vi "Process0.vi"(9 "process sync":refnum<notifier>, 11 "Main in":refnum<class "Main.lvclass">) -> ()   [LabVIEW 2019, in "Main.lvclass"]
doc: "Developed by Kevin Thompson\nkevin@thompsonengineering.net\n\nCopyright 2018\nThompson Engineering, LLC"
uses:
  Main.lvclass
  <vilib>/TELLC/SMQ/Add States to Queue using MultiLine String with vData.vi
  DataTypes/Process - AppData--cluster.ctl
  Common/DataTypes/TD Async CmdMsg EventData--cluster.ctl
  DataTypes/Public Events--cluster.ctl
  DataTypes/Dependency--cluster.ctl
  DataTypes/Settings--cluster.ctl
  Log_Engine/Log_Engine.lvclass
  DAQ_Engine/DAQ_Engine.lvclass
  Config/Config.lvclass
  Common/DataTypes/RawChannelData--cluster.ctl
  Common/DataTypes/RawDAQData--cluster.ctl
  Common/DataTypes/ChannelWaveforms--cluster.ctl
  Common/DataTypes/InverterWaveforms--cluster.ctl
  Common/DataTypes/InverterWaveforms--QRef.ctl
  Common/DataTypes/RawDAQDataQRef--cluster.ctl
  support/Data Algorithms/subvis/DataTypes/averaging variables.ctl
  support/Data Algorithms/subvis/DataTypes/ESR alarm variables.ctl
  support/Data Algorithms/subvis/DataTypes/Processing loop variables--cluster.ctl
  DataTypes/PrivateAsynEv_Main--enum.ctl
  Common/DataTypes/Measurement Config--cluster.ctl
  Common/DataTypes/DAQState--enum.ctl
  Common/DataTypes/Acquisition Mode--cluster.ctl
  support/Data Algorithms/subvis/DataTypes/Gain control.ctl
  Common/DataTypes/TDMSState--enum.ctl
  Common/DataTypes/LogState--enum.ctl
  Common/DataTypes/UpdateControlValue EvData--cluster.ctl
  support/Data Algorithms/subvis/DataTypes/ESR scaling--cluster.ctl
  DataTypes/DataProcessAuxData--cluster.ctl
  Common/DataTypes/DataProcAuxDat--Qref.ctl
  DataTypes/ProcessingState--enum.ctl
  DataTypes/ProcessingStateChg EvData--cluster.ctl
  DataTypes/InverterInfo--cluster.ctl
  DataTypes/ProcessInitParams--cluster.ctl
  DataTypes/StartProcInitParams--cluster.ctl
  Common/DataTypes/inverter offset range--cluster.ctl
  Common/DataTypes/inverter gain range--cluster.ctl
  Common/DataTypes/inverter info v2--cluster.ctl
  Common/DataTypes/Inverter database record v2--cluster.ctl
panel:
  in  "Data Rate 9775(S/s)":dbl=3.0 format="%#.6p"
  out "DAQ data":T1
  out "RawDaqDataQ size":i32
  in  "reset averaging":bool
  in  "Dummy Vrms":dbl=120.0
  in  "UseDummyVrms":bool
  in  "ESR scaling":T3[](array[typedef])
  in  "Data Rate 9215 (S/s)":dbl=1200000.0 format="%#.6p"
  in  "Settings.Signal scaling":T4[](array[typedef])
  in  "Exit":bool
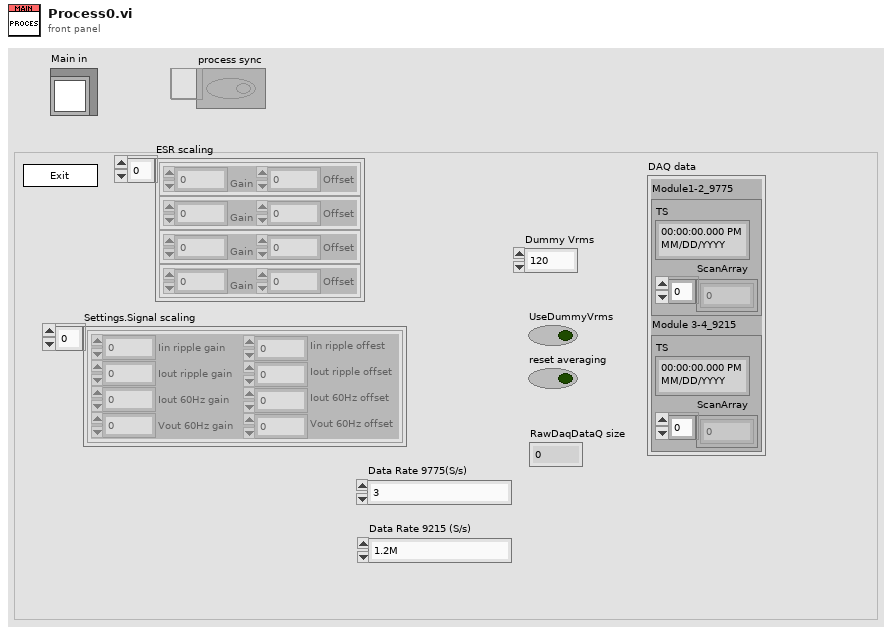
[diagram p1: front panel]
types:
  T1 = typedef "RawDAQData--cluster.ctl" = cluster{"Module1-2_9775":T2, "Module 3-4_9215":T2}
  T2 = typedef "RawChannelData--cluster.ctl" = cluster{"TS":timestamp, "ScanArray":dbl[]}
  T3 = typedef "Main.lvclass/ESR scaling--cluster.ctl" = cluster{"Gain":dbl, "Offset":dbl}
  T4 = typedef "Main.lvclass/Gain control.ctl" = cluster{"Iin ripple gain":dbl, "Iout ripple gain":dbl, "Iout 60Hz gain ":dbl, "Vout 60Hz gain ":dbl, "Iin ripple offest":dbl, "Iout ripple offset":dbl, "Iout 60Hz offset":dbl, "Vout 60Hz offset":dbl}
  T5 = typedef "Main.lvclass/Processing loop variables--cluster.ctl" = cluster{"DUT ESR avg":T6[], "DUT  PF avg":T6[], "DUT  Power avg ":T6[], "DUT processed data":cluster{"raw ESR":dbl, "Tcomp, avg ESR":dbl, "Vout RMS":dbl, "Iout RMS":dbl, "power factor":dbl, "power":dbl, "efficiency":dbl}[], "ESR alarm variables":T7[], "Status data":cluster{"Inv. 1 on?":bool, "Inv. 1 ESR over threshhold?":bool, "Minimum current":dbl}[], "CurrInverter":T8[], "miscellaneous":cluster{"Inverter 1 ID":string, "Inverter 2 ID":string, "Packet count":u32, "Calibration":dbl, "Calibration Gain":dbl, "Calibration Offset":dbl, "Calculated Total Power":dbl, "Seconds":dbl, "Last Tag Event":dbl, "Tag Event Time":dbl}[], "DUT INVERTER data":cluster{"Raw ESR sum":dbl, "scaled raw ESR sum":dbl, "scaled and averaged raw ESR sum":dbl, "Total power":dbl}[]}
  T6 = typedef "Main.lvclass/averaging variables.ctl" = cluster{"raw value buffer":dbl[], "buffer index":i32, "Avg value":dbl, "num to avg":i32}
  T7 = typedef "Main.lvclass/ESR alarm variables.ctl" = cluster{"Inv 1 baseline ESR":dbl, "Inv 1 over threshold?":bool, "Alarm on?":bool, "inv 1 esr chart range":dbl, "inv 1 esr saved baseline":dbl, "ESR alarm threshhold":dbl}
  T8 = typedef "Inverter database record v2--cluster.ctl" = cluster{"name":string, "last updated":timestamp, "type":string, "inverter Info":T9, "gain range":T10, "offset range":T11, "gain actual":dbl, "offset actual":dbl, "power level":dbl, "minimum current":dbl, "resistance single phase":dbl, "resistance 3 phase":dbl, "set flag":u16}
  T9 = typedef "inverter info v2--cluster.ctl" = cluster{"manufacturer":string, "model":string, "product":string, "serial":string, "power class":string, "year manf":string}
  T10 = typedef "inverter gain range--cluster.ctl" = cluster{"gain max":dbl, "gain min":dbl, "gain increment":dbl}
  T11 = typedef "inverter offset range--cluster.ctl" = cluster{"offset max":dbl, "offset min":dbl, "offset increment":dbl}
  T12 = typedef "InverterWaveforms--cluster.ctl" = T13[]
  T13 = typedef "ChannelWaveforms--cluster.ctl" = cluster{"Iin ripple ":waveform(dbl), "Iout ripple ":waveform(dbl), "Iout 60Hz":waveform(dbl), "Vout 60Hz":waveform(dbl)}
  T14 = typedef "Main.lvclass/ProcessingState--enum.ctl" = enum16{"Idle", "Starting", "Running", "Done", "Error"}
  T15 = typedef "Main.lvclass/Process - AppData--cluster.ctl" = cluster{"Core":cluster{"Current VI Reference":refnum<vi>, "Close Panel on Exit?":bool}, "Your Boolean data":bool, "Your string data":string, "SMQ":refnum<queue>, "Initialized?":bool, "Self Reference":refnum<class "Main.lvclass">, "Simulation?":bool, "process sync":refnum<notifier>, "vData":variant, "Settings":T16, "Dependency":T17, "Public Events":T18, "RawDaqDataQ":T19, "InverterWaveformsQ":T20, "Processing loop variables":T5, "Measurement config":T21, "Acquisition mode":T22, "DAQState":T23, "Signal scaling":T4, "PrivateAsync Ev":refnum<user-event>, "LogState":T24, "TDMSState":T25, "InvWfmsQ-DT":T20, "DPAuxDataQ":T26, "ProcessingState":T14, "InverterInfo":T27, "ProcLoopInterval":u32, "StoredESR Baseline":dbl, "StoreESR BLine Flag":bool, "UseSavedESR BLine Flag":bool}
  T16 = typedef "Main.lvclass/Settings--cluster.ctl" = cluster{"Simulation":bool, "Signal scaling":T4[], "ESR scaling":T3[], "num readings to average":i32[], "ESR alarm threshhold (%)":i32[], "UseDummyVrms":bool, "Dummy Vrms":dbl, "Inverter Database File":path, "default Inverter (name)":string[]}
  T17 = typedef "Main.lvclass/Dependency--cluster.ctl" = cluster{"Config":refnum<class "Config.lvclass">, "DAQ":refnum<class "DAQ_Engine.lvclass">, "Log_Engine":refnum<class "Log_Engine.lvclass">}
  T18 = typedef "Main.lvclass/Public Events--cluster.ctl" = cluster{"Main.AsyncCmd Event":refnum<user-event>, "Main.AsyncMsg Event":refnum<user-event>, "stop process":refnum<user-event>, "UpdateControlValue Ev":refnum<user-event>, "ProcessingStateChg Ev":refnum<user-event>}
  T19 = typedef "RawDAQDataQRef--cluster.ctl" = refnum<queue>
  T20 = typedef "InverterWaveforms--QRef.ctl" = refnum<queue>
  T21 = typedef "Measurement Config--cluster.ctl" = cluster{"Data Rate 9775":dbl, "Data Rate 9215":dbl, "Samples RMS 9215":u32, "Samples RMS 9775":u32}
  T22 = typedef "Acquisition Mode--cluster.ctl" = enum16{"3phase", "Single"}
  T23 = typedef "DAQState--enum.ctl" = enum16{"Unknown", "Stopped", "Running", "Error"}
  T24 = typedef "LogState--enum.ctl" = enum16{"Unknown", "Stopped", "Running", "Error"}
  T25 = typedef "TDMSState--enum.ctl" = enum16{"Unknown", "Stopped", "Running", "Error"}
  T26 = typedef "DataProcAuxDat--Qref.ctl" = refnum<queue>
  T27 = typedef "InverterInfo--cluster.ctl" = cluster{"Inverter ID":string}
  T28 = typedef "Main.lvclass/ObjData--cluster.ctl" = cluster{"Settings":T16, "Public Events":T18, "Dependency":T17, "ReadData-placeholder":T29, "VISA-placeholder":refnum<visa-resource-name>, "InverterWaveformsQ":T20, "Application.TerminateProcess Event":refnum<user-event>, "RawDaqDataQ":T19, "MeasSettings":T21, "InverterDataAcqMode":T22, "DAQState Data":T30, "Private Events":T31, "InvWfmsQ-DT":T20, "DPAuxDataQ":T26, "ProcessingState":T14, "InverterInfo":T27, "CurrInverters":T8[], "InverterLUT Dict":T32, "ESR Chart Ref":refnum<vi>, "StoreESR BLine Ref":refnum<vi>, "UseSavedESR BLine Ref":refnum<vi>}
  T29 = typedef "Main.lvclass/Read Data--cluster.ctl" = cluster{"Data":dbl}
  T30 = typedef "DAQ_Engine.lvclass/DAQStateEvData--cluster.ctl" = cluster{"DAQState":T23, "vData":variant}
  T31 = typedef "Main.lvclass/Private Events--cluster.ctl" = cluster{"PrivateAsync Ev":refnum<user-event>}
  T32 = typedef "TD Dynamic CVT DVR--ref.ctl" = refnum<data-value>
  T33 = enum16{"Event Loop -", "Async Loop -", "DataProc Loop - "}
  T34 = typedef "Main.lvclass/PrivateAsynEv_Main--enum.ctl" = enum16{"PrivMain.UpdateMeasSettings", "PrivMain.UpdateAcqMode", "PrivMain.UpdateDAQState", "PrivMain.UpdateLogState", "PrivMain.UpdateTDMSState", "PrivMain.UpdateProcessingState", "PrivMain.Stop&Terminate", "PrivMain.CurrInverterUpdated", "PrivMain.UpdateStoreUseESRBaseline", "PrivMain.SetUnsetAlarm&ESRBLine", "PrivMain.ResetAveraging"}
  T35 = cluster{"VoltageDyn":dbl, "CurrentDyn":dbl, "MotorV SP":dbl}[]
  T36 = typedef "DataProcessAuxData--cluster.ctl" = cluster{"Time Stamp":timestamp, "Raw ESR sum":dbl, "Inv 1 ON?":bool, "Average scaled ESR sum":dbl, "Inv 1 over threshold?":bool, "Inv 1 ESR":cluster{"ESR Baseline":dbl, "Alarm threshhold (%)":dbl, "Avg value":dbl}, "Max ESR":dbl}
  T37 = typedef "TD MeasData--cluster.ctl" = cluster{"Timestamp":timestamp, "ESR_Ohm":dbl[], "DUT data":T38[], "DUT INVERTER data":cluster{"Raw ESR sum":dbl, "scaled raw ESR sum":dbl, "scaled and averaged raw ESR sum":dbl, "Total power":dbl}[]}
  T38 = typedef "InverterPhaseData--cluster.ctl" = cluster{"RawESR_Ohm":dbl, "TcompAvgESR_Ohm":dbl, "VoutRMS_V":dbl, "IoutRMS_A":dbl, "PF":dbl, "AvgPF":dbl, "Power_W":dbl, "AvgPower_W":dbl, "efficiency":dbl}
  T39 = enum32{"invalid app kind", "Development System", "Run Time System", "Student Edition", "Embedded LabVIEW", "Evaluation", "Custom"}
  T40 = enum32{"Invalid", "Standard", "Closed", "Hidden", "Minimized", "Maximized"}
  T41 = cluster{"Inv. 1 on?":bool, "Inv. 1 ESR over threshhold?":bool, "Minimum current":dbl}
  T42 = cluster{"Inverter 1 ID":string, "Inverter 2 ID":string, "Packet count":u32, "Calibration":dbl, "Calibration Gain":dbl, "Calibration Offset":dbl, "Calculated Total Power":dbl, "Seconds":dbl, "Last Tag Event":dbl, "Tag Event Time":dbl}
  T43 = typedef "Main.lvclass/AsynCmd_Main--enum.ctl" = enum16{"Main.StartProcessing", "Main.StopProcessing", "Main.RefreshInverterList"}
  T44 = typedef "Main.lvclass/StartProcInitParams--cluster.ctl" = cluster{"InverterInfo":T27, "ProcessInitParams":T45}
  T45 = typedef "Main.lvclass/ProcessInitParams--cluster.ctl" = cluster{"MinCurrThreshold":dbl, "NumPF RdsToAvg":i32, "ESR alarm threshhold (%)":dbl, "# readings to average":i32}
  T46 = typedef "Main.lvclass/AsynMsg_Main--enum.ctl" = enum16{"Main.CurrInverterUpdated"}
  T47 = typedef "DAQ_Engine.lvclass/DAQMeasSettingsEvData--cluster.ctl" = cluster{"Measurement config":T21, "vData":variant}
  T48 = typedef "Log_Engine.lvclass/LogStateEvData--cluster.ctl" = cluster{"LogState":T24, "vData":variant}
  T49 = typedef "Log_Engine.lvclass/TDMSStateEvData--cluster.ctl" = cluster{"TDMSState":T25, "vData":variant}
  T50 = typedef "DAQ_Engine.lvclass/Public Events--cluster.ctl" = cluster{"DAQ_Engine.AsyncCmd Event":refnum<user-event>, "DAQ_Engine.AsyncMsg Event":refnum<user-event>, "stop process":refnum<user-event>, "DAQ_Engine.DAQStateChg Ev":refnum<user-event>, "DAQ_Engine.MeasSettingsChg Ev":refnum<user-event>, "DAQ_Engine.AcqModeChg Ev":refnum<user-event>}
  T51 = typedef "Log_Engine.lvclass/Public Events--cluster.ctl" = cluster{"Log_Engine.AsyncCmd Event":refnum<user-event>, "Log_Engine.AsyncMsg Event":refnum<user-event>, "stop process":refnum<user-event>, "Log_Engine.LogStateChg Ev":refnum<user-event>, "Log_Engine.TDMSStateChg Ev":refnum<user-event>}
  T52 = cluster{"Current VI Reference":refnum<vi>, "Close Panel on Exit?":bool}
  T53 = cluster{"ProcessingState":T14, "Variant":variant}
  T54 = cluster{"Inv. 1 on?":bool, "Inv. 1 ESR over threshhold?":bool, "Minimum current":dbl}[]
  T55 = cluster{"Inverter 1 ID":string, "Inverter 2 ID":string, "Packet count":u32, "Calibration":dbl, "Calibration Gain":dbl, "Calibration Offset":dbl, "Calculated Total Power":dbl, "Seconds":dbl, "Last Tag Event":dbl, "Tag Event Time":dbl}[]
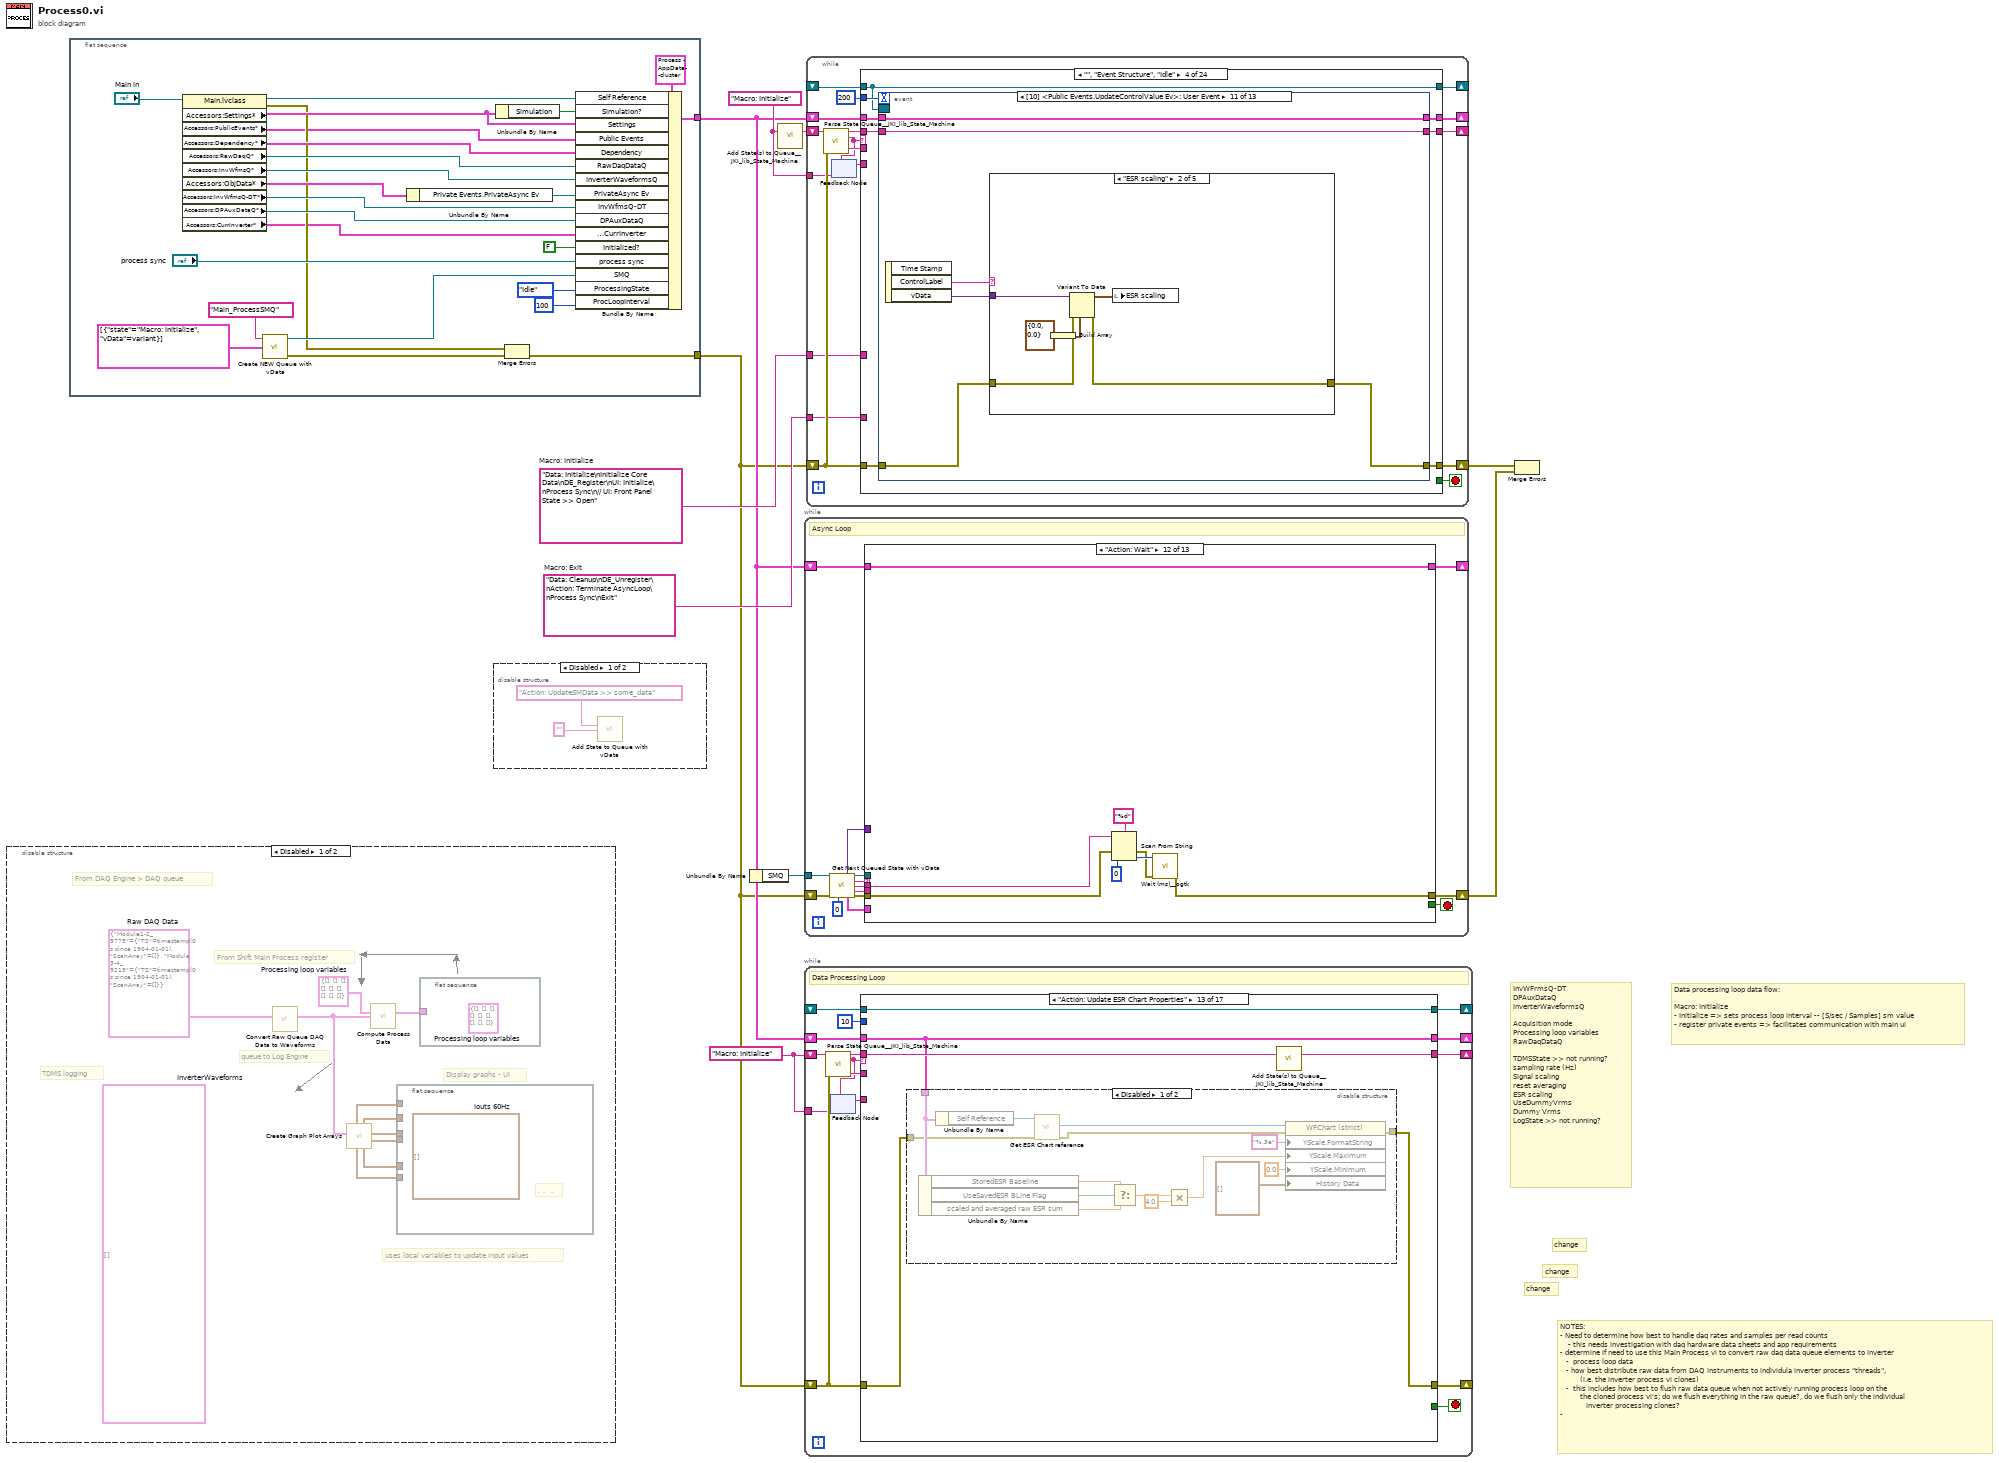
[diagram p0: block diagram]
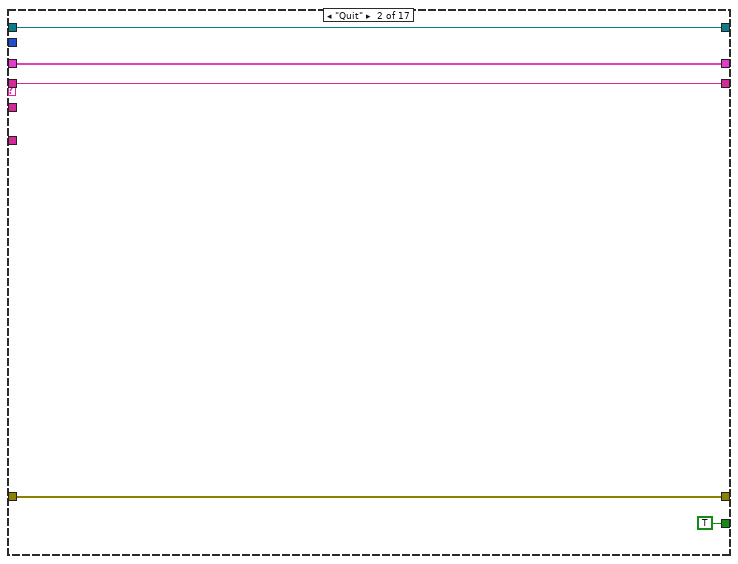
[diagram p4: hidden frame]
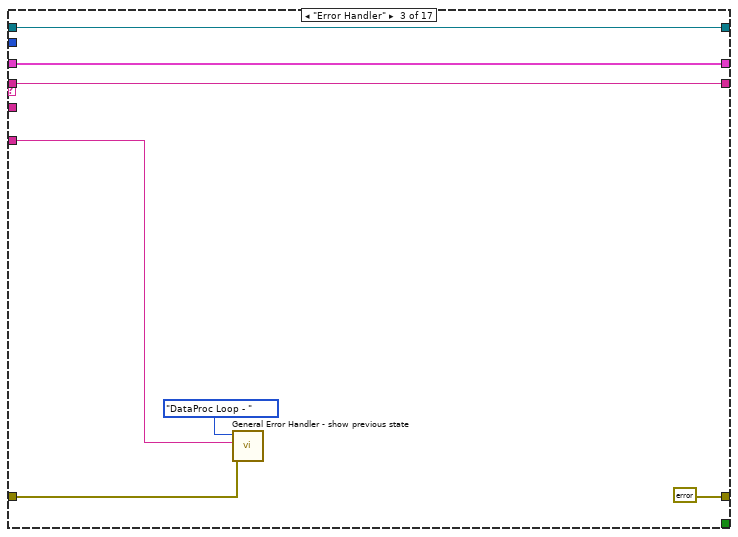
[diagram p5: hidden frame]
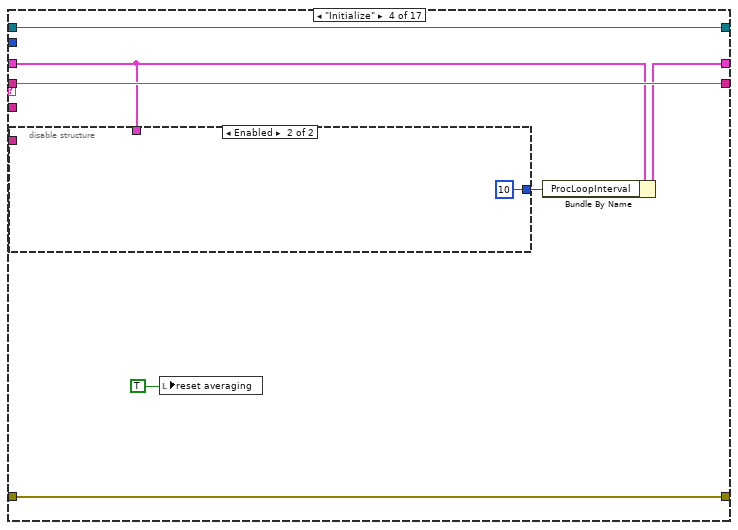
[diagram p6: hidden frame]
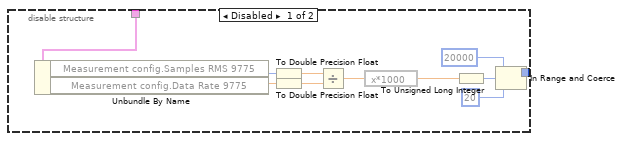
[diagram p7: hidden frame]
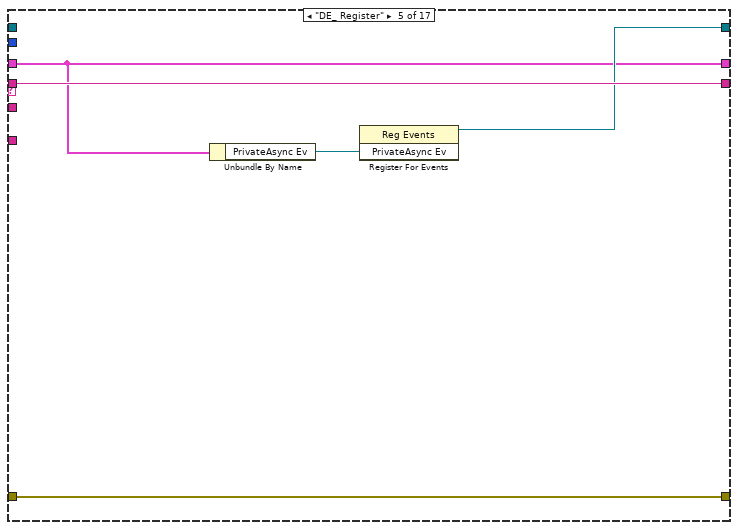
[diagram p8: hidden frame]
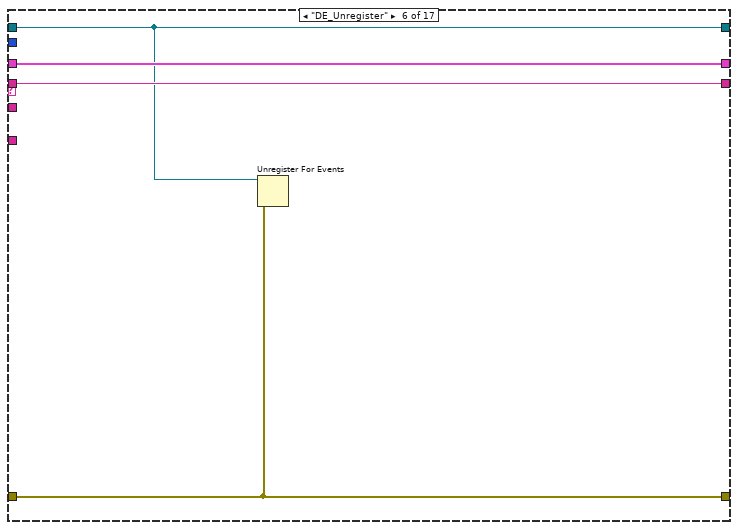
[diagram p9: hidden frame]
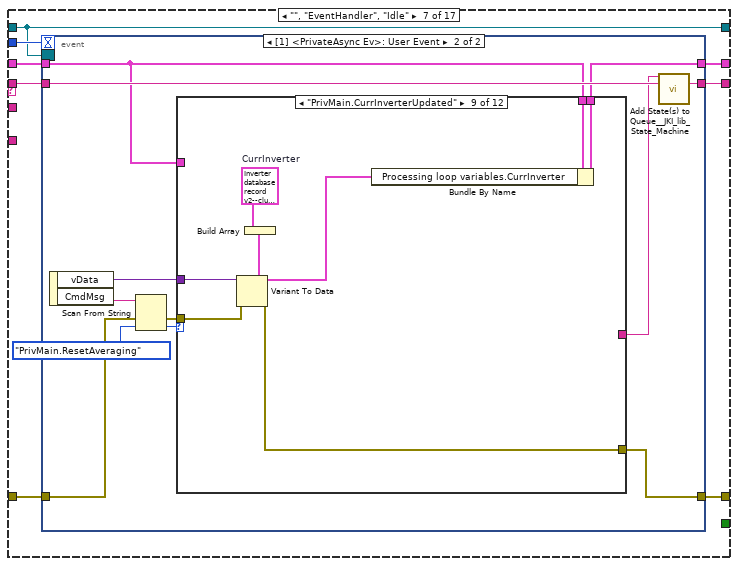
[diagram p10: hidden frame]
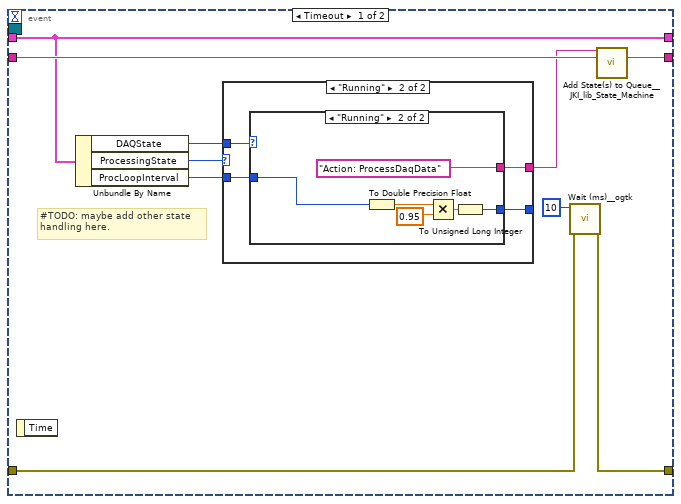
[diagram p11: hidden frame]
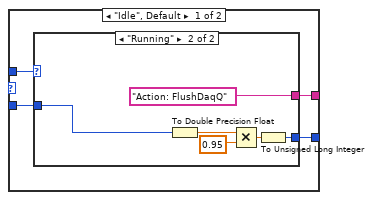
[diagram p12: hidden frame]
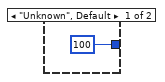
[diagram p13: hidden frame]
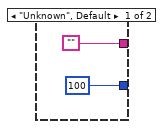
[diagram p14: hidden frame]
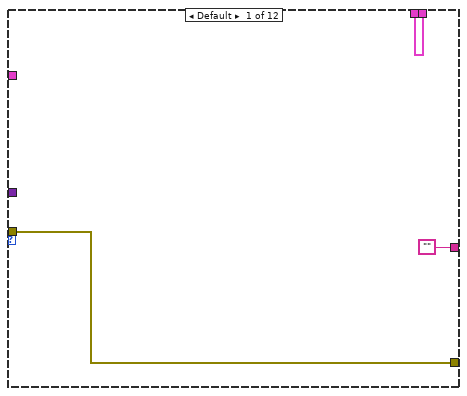
[diagram p15: hidden frame]
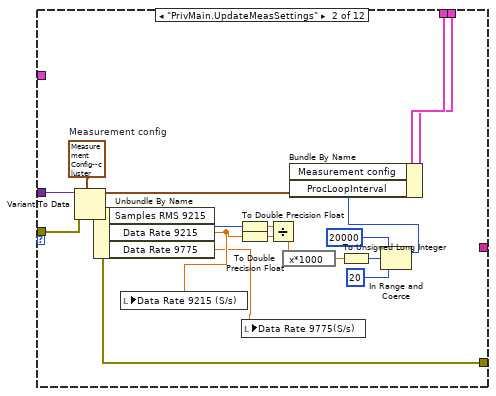
[diagram p16: hidden frame]
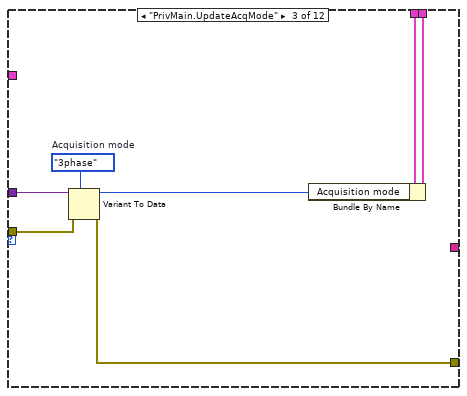
[diagram p17: hidden frame]
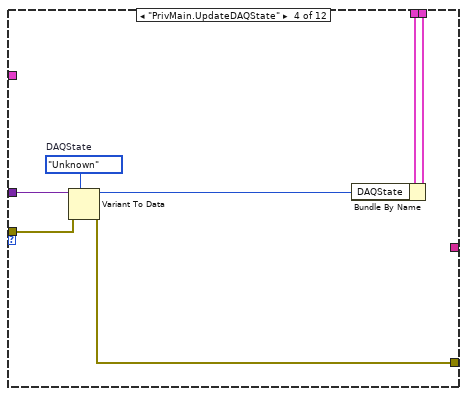
[diagram p18: hidden frame]
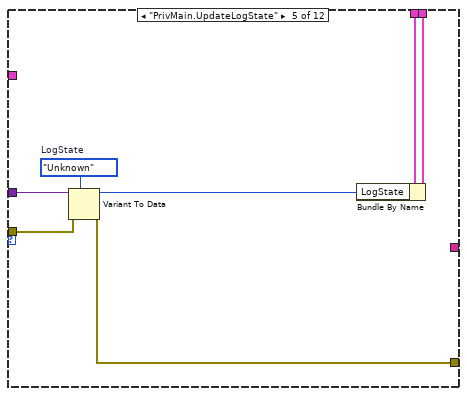
[diagram p19: hidden frame]
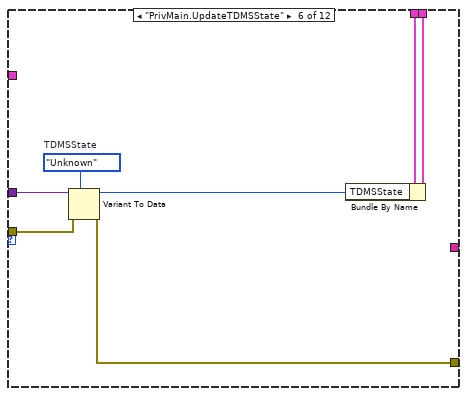
[diagram p20: hidden frame]
diagram:
  w1 = "Macro: Initialize"
  w8 = "Data: Cleanup\nDE_Unregister\nAction: Terminate AsyncLoop\nProcess Sync\nExit"  # Macro: Exit
  w9 = "Data: Initialize\nInitialize Core Data\nDE_Register\nUI: Initialize\nProcess Sync\n// UI: Front Panel State >> Open"  # Macro: Initialize
  w4 = "Macro: Initialize"
  # "change"
  # "change"
  # "change"
  # "NOTES:\n- Need to determine how best to handle daq rates and samples per read counts\n    - this needs investigation with daq hardware data sheets and app requirements\n- determine if need to use this Main Process vi to convert raw daq data queue elements to inverter\n   -  process loop data\n   - how best distribute raw data from DAQ instruments to individula inverter process \"threads\",\n          (i.e. the inverter process vi clones)\n   -  this includes how best to flush raw data queue when not actively running process loop on the\n          the cloned process vi's; do we flush everything in the raw queue?, do we flush only the individual\n             inverter processing clones?\n-"
  # "Data processing loop data flow:\n\nMacro: Initialize\n- Initialize => sets process loop interval -- [S/sec / Samples] sm value\n- register private events => facilitates communication with main ui"
  # "InvWFrmsQ-DT\nDPAuxDataQ\nInverterWaveformsQ\n\nAcquisition mode\nProcessing loop variables\nRawDaqDataQ\n\nTDMSState >> not running?\nsampling rate (Hz)\nSignal scaling\nreset averaging\nESR scaling\nUseDummyVrms\nDummy Vrms\nLogState >> not running?"
  n1 = disable-structure shown="Disabled" {
    frame Disabled {
      w12 = T5 {"DUT ESR avg"=[], "DUT  PF avg"=[], "DUT  Power avg "=[], "DUT processed data"=[], "ESR alarm variables"=[], "Status data"=[], "CurrInverter"=[], "miscellaneous"=[], "DUT INVERTER data"=[]}  # Processing loop variables
      (unwired) T12 []  # InverterWaveforms
      w13 = T1 {"Module1-2_9775"={"TS"=timestamp(0 s since 1904-01-01), "ScanArray"=[]}, "Module 3-4_9215"={"TS"=timestamp(0 s since 1904-01-01), "ScanArray"=[]}}  # Raw DAQ Data
      # "uses local variables to update input values"
      # "queue to Log Engine"
      # "From Shift Main Process register"
      # "From DAQ Engine > DAQ queue"
      # "TDMS logging"
      # "Display graphs - UI"
      n2 = call "Convert Raw Queue DAQ Data to Waveforms.vi"("RawDAQData in"=w13) -> ("InverterWaveforms out"=w14:T12)  [unwired: 9 in, 1 out]
      n3 = call "Create Graph Plot Arrays.vi"("InverterWaveforms"=w14) -> ("DUT1 60 Hz V and I"=w20:waveform(dbl)[], "Iouts 60Hz"=w17:waveform(dbl)[], "DUT2 60 Hz V and I"=w19:waveform(dbl)[], "Iout ripples"=w16:waveform(dbl)[], "DUT3 60 Hz V and I"=w18:waveform(dbl)[], "Iin ripples"=w15:waveform(dbl)[])  [unwired: 3 in, 2 out]
      n4 = call "Compute Process Data.vi"("Processing loop variables"=w12, "InverterWaveforms"=w14) -> ("Processing loop vars out"=w11:T5)  [unwired: 10 in, 3 out]
      n5 = flat-sequence {
        tunnel: w20 -> [_]
        tunnel: w19 -> [_]
        tunnel: w18 -> [_]
        tunnel: w17 -> [_]
        tunnel: w16 -> [_]
        tunnel: w15 -> [_]
        frame #0 {
          (unwired) waveform(dbl)[] []  # Iouts 60Hz
          # ".  .   ."
        }
      }
      n6 = flat-sequence {
        tunnel: w11 -> [_]
        frame #0 {
          (unwired) T5 {"DUT ESR avg"=[], "DUT  PF avg"=[], "DUT  Power avg "=[], "DUT processed data"=[], "ESR alarm variables"=[], "Status data"=[], "CurrInverter"=[], "miscellaneous"=[], "DUT INVERTER data"=[]}  # Processing loop variables
        }
      }
    }
    frame Enabled {
    }
  }
  n7 = flat-sequence {
    tunnel: [w45] -> w3
    tunnel: [w26] -> w2
    frame #0 {
      n8 = property class="Main.lvclass"(reference="Main in") -> (reference out=w24:refnum<class "Main.lvclass">, error out=w25:errorcluster, "Accessors:Settings*"=w36:T16, "Accessors:PublicEvents*"=w23:T18, "Accessors:Dependency*"=w38:T17, "Accessors:RawDaqQ*"=w34:T19, "Accessors:InvWfmsQ*"=w33:T20, "Accessors:ObjData*"=w32:T28, "Accessors:InvWfmsQ-DT*"=w30:T20, "Accessors:DPAuxDataQ*"=w29:T26, "Accessors:CurrInverter*"=w21:T8[])  [unwired: 1 in]
      n9 = call <vilib>:"Create NEW Queue with vData.vi"("Initial States"=cluster{"state":string, "vData":variant}[] [{"state"="Macro: Initialize", "vData"=variant}], "Name (SMQ)"="Main_ProcessSMQ") -> ("error out"=w42:errorcluster, "queue out"=w44:refnum<queue>)  [unwired: 2 in]
      n10 = Unbundle By Name(w32) -> ("Private Events.PrivateAsync Ev"=w31:refnum<user-event>)
      n11 = Unbundle By Name(w36) -> ("Simulation"=w37:bool)
      n12 = Merge Errors(w25, w42) -> (w26:errorcluster)
      n13 = Bundle By Name(cluster=T15 {"Core"={"Current VI Reference"=refnum, "Close Panel on Exit?"=FALSE}, "Your Boolean data"=FALSE, "Your string data"="", "SMQ"=refnum, "Initialized?"=FALSE, "Self Reference"=refnum, "Simulation?"=FALSE, "process sync"=refnum, "vData"=variant, "Settings"={"Simulation"=FALSE, "Signal scaling"=[], "ESR scaling"=[], "num readings to average"=[], "ESR alarm threshhold (%)"=[], "UseDummyVrms"=FALSE, "Dummy Vrms"=0.0, "Inverter Database File"=path "", "default Inverter (name)"=[]}, "Dependency"={"Config"=refnum, "DAQ"=refnum, "Log_Engine"=refnum}, "Public Events"={"Main.AsyncCmd Event"=refnum, "Main.AsyncMsg Event"=refnum, "stop process"=refnum, "UpdateControlValue Ev"=refnum, "ProcessingStateChg Ev"=refnum}, "RawDaqDataQ"=refnum, "InverterWaveformsQ"=refnum, "Processing loop variables"={"DUT ESR avg"=[], "DUT  PF avg"=[], "DUT  Power avg "=[], "DUT processed data"=[], "ESR alarm variables"=[], "Status data"=[], "CurrInverter"=[], "miscellaneous"=[], "DUT INVERTER data"=[]}, "Measurement config"={"Data Rate 9775"=3.0, "Data Rate 9215"=1200000.0, "Samples RMS 9215"=480000, "Samples RMS 9775"=3}, "Acquisition mode"=enum."3phase", "DAQState"=enum."Unknown", "Signal scaling"={"Iin ripple gain"=13.333, "Iout ripple gain"=13.333, "Iout 60Hz gain "=14.286, "Vout 60Hz gain "=20.0, "Iin ripple offest"=0.0, "Iout ripple offset"=0.0, "Iout 60Hz offset"=0.0, "Vout 60Hz offset"=0.0}, "PrivateAsync Ev"=refnum, "LogState"=enum."Unknown", "TDMSState"=enum."Unknown", "InvWfmsQ-DT"=refnum, "DPAuxDataQ"=refnum, "ProcessingState"=enum."Idle", "InverterInfo"={"Inverter ID"=""}, "ProcLoopInterval"=0, "StoredESR Baseline"=0.0, "StoreESR BLine Flag"=FALSE, "UseSavedESR BLine Flag"=FALSE} ("SM2 AppData"), "Self Reference"=w24, "Simulation?"=w37, "Settings"=w36, "Public Events"=w23, "Dependency"=w38, "RawDaqDataQ"=w34, "InverterWaveformsQ"=w33, "PrivateAsync Ev"=w31, "InvWfmsQ-DT"=w30, "DPAuxDataQ"=w29, "Processing loop variables.CurrInverter"=w21, "Initialized?"=FALSE, "process sync"="process sync", "SMQ"=w44, "ProcessingState"=ProcessingState--enum."Idle", "ProcLoopInterval"=u32 100) -> (w45:T15)
    }
  }
  n14 = disable-structure shown="Disabled" {
    frame Disabled {
      n15 = call <vilib>:"Add State to Queue with vData.vi"("state in"="Action: UpdateSMData >> some_data", "vData (\"\")"="") -> ()  [unwired: 10 in, 4 out]
    }
    frame Enabled {
    }
  }
  n16 = Unbundle By Name(w3) -> ("SMQ"=w7:refnum<queue>)
  n17 = call <vilib>:"Add State(s) to Queue__JKI_lib_State_Machine.vi"("State(s) in (\"\")"=w4) -> ("States Out"=w10:string)  [unwired: 14 in]
  n18 = while {
    shift-right: [w58] -> w5
    shift-left: w2 -> [w60]
    tunnel: w7 -> [w56]
    shift-right: [w54] -> _
    shift-left: w3 -> [w55]
    stop <- w49 stop-if-true
    # "Async Loop"
    n19 = call <vilib>:"Get Next Queued State with vData.vi"("queue in"=w56, "error in (no error)"=w60, "timeout (100)"=0) -> ("vData out"=w53:variant, "queue out"=w57:refnum<queue>, "Next State"=w61:string, "queued msg"=w51:string, "Prev State"=w50:string, "RemainingElements"=w48:cluster{"state":string, "vData":variant}[], "error out"=w59:errorcluster)  [unwired: 6 in]
    n20 = case shown="\"Action: Wait\"" w61 {
      tunnel: w57 -> [_ _ _ _ w80 w90 _ w106 w111 _ _ _ w148]
      tunnel: w51 -> [_ _ _ _ _ _ _ _ _ _ _ w137 w150]
      selector: w61 -> [w62 _ _ _ _ _ _ _ _ _ _ _ _]
      tunnel: w59 -> [w64 w72 w74 w79 w86 w88 w102 w105 w110 w114 w116 w136 w145]
      tunnel: [w63 w72 errorcluster {"status"=FALSE, "code"=0, "source"=""} ("error constant") w79 w86 w87 w102 w104 w109 w114 w116 w139 w144] -> w58
      tunnel: w55 -> [w70 w71 w77 w78 w85 w89 w101 w107 w112 w113 w117 w142 w147]
      tunnel: [w70 w71 w77 w78 w85 w89 w101 w107 w112 w113 w117 w142 w146] -> w54
      tunnel: w53 -> [_ _ _ _ _ _ _ _ _ _ _ _ w149]
      tunnel: w50 -> [_ _ w73 _ _ _ _ _ _ _ _ _ _]
      tunnel: [_ _ _ _ TRUE _ _ _ _ _ _ _ _] -> w49
      tunnel: w48 -> [_ _ _ _ _ _ _ _ _ _ _ _ _]
      frame Default {
        w66 = 42 items=["No error", "Argument error", "Memory is full", "Out of zone", "End of file", "File already open", "Generic file I/O error", "File not found", "File permission error", "Disk is full", "Duplicate path", "Too many files open", "System feature not enabled", "Resource file not found", "Cannot add resource", "Resource not found", "Image not found", "Image memory error", "Pen does not exist", "Config type invalid", "Config token not found", "Config parse error", "Config memory error", "Bad external code format", "Bad external code offset", "External code not present", "Null window", "Destroy window error", "Null menu", "Print aborted", "Bad print record", "Print driver error", "Windows error during printing", "Memory error during printing", "Print dialog error", "Generic print error", "Invalid device refnum", "Device not found", "Device parameter error", "Device unit error", "Cannot open device", "Device call aborted", "Generic error", "Cancelled by user", "Object ID too low", "Object ID too high", "Object not in heap", "Unknown heap", "Unknown object (invalid DefProc)", "Unknown object (DefProc not in table)", "Message out of range", "Invalid (null) method", "Unknown message", "Manager call not supported", "Bad address", "Network operation in progress", "Network operation timed out", "Connection is busy", "Network attribute not supported", "Network error", "Address in use", "System out of memory", "Connection aborted", "Connection refused", "Not connected", "Already connected", "Connection closed", "Initialization error (interapplication manager)", "Bad occurrence", "Wait on unbound occurrence handler", "Occurrence queue overflow", "Datalog type conflict", "Unused", "Unrecognized type (interapplication manager)", "Memory corrupt", "Failed to make temporary DLL", "Old CIN version", "Drag socket not found", "Failed to load drop-object", "Failed to register OLE object", "Failed to release OLE object", "Format specifier type mismatch", "Unknown format specifier", "Too few format specifiers", "Too many format specifiers", "Scan failed", "Newer CIN version", "Error converting to variant", "Runtime menu error", "Password tampered", "Variant attribute not found", "Incompatible variant data type", "Event data is not available", "Event Store is not present", "Occurrence is not found", "Event Queue is not created", "Event info is not available", "Refnum passed is NULL", "Error retrieving Class GUID", "Error retrieving CoClass GUID", "Error retrieving TypeLib GUID.", "Bad built application magic bytes.", "Specific driver is different from the specific driver associated with the Logical Name.", "There is no session opened to the class driver.", "Max Error", "MAX - Error with config objects", "MAX - Error loading configuration", "MAX - Group not supported"]
        n21 = Format Into String(format string="Software Exception: Unhandled State \"%s\"." ("message"), error in=w64, w62) -> (resulting string=w67:string, error out=w68:errorcluster)  [unwired: 1 in]
        n22 = call <vilib>:"Error Cluster From Error Code.vi"("show call chain? (False)"=TRUE, "error in (no error)"=w68, "error message (\"\")"=w67, "error code (0)"=w66) -> ("error out"=w63:errorcluster)  [unwired: 5 in]
      }
      frame "Initialize" {
      }
      frame "Error Handler" {
        n23 = call "General Error Handler - show previous state.vi"("error in (no error)"=w74, "Previous State"=w73, "Loop Select"=enum16{"Event Loop -", "Async Loop -"}."Async Loop -") -> ()  [unwired: 7 in, 2 out]
      }
      frame "CleanUp" {
      }
      frame "Exit" {
        n24 = Flush Queue(queue=w80) -> (queue out=w83:refnum<queue>, error out=w82:errorcluster)  [unwired: 1 in, 1 out]
        n25 = Release Queue(queue=w83, force destroy? (F)=TRUE, error in (no error)=w82) -> ()  [unwired: 3 out]
      }
      frame "", "Idle" {
        # "#NOTE: This Async Loop NOT USED in this app.\nNeeded faster response; see bottom loop.\nCode remains here for reference and re-use if needed."
        # "#TODO: add condition"
        n26 = Unbundle By Name(w89) -> ()  [unwired: 1 out]
        n27 = case shown="False" FALSE {
          tunnel: w90 -> [_ w100]
          tunnel: w88 -> [w93 w97]
          tunnel: [w92 w95] -> w87
          frame False {
            n28 = call <userlib>:"Wait (ms)__ogtk.vi"("error in (no error)"=w93, "milliseconds to wait"=u32 200) -> ("error out"=w92:errorcluster)  [unwired: 8 in, 1 out]
          }
          frame True {
            n29 = call <userlib>:"Wait (ms)__ogtk.vi"("error in (no error)"=w97, "milliseconds to wait"=u32 50) -> ("error out"=w98:errorcluster)  [unwired: 8 in, 1 out]
            n30 = call-poly <vilib>:"Polymorphic - Add States(s) To Queue.vi"("queue in"=w100, "state in"="Action: ReadRawDaqQueue", "error in"=w98) -> ("error out"=w95:errorcluster)  [unwired: 9 in, 3 out]
          }
        }
      }
      frame "------ Macro ------" {
      }
      frame "Macro: Initialize" {
        n31 = call-poly <vilib>:"Polymorphic - Add States(s) To Queue.vi"("queue in"=w106, "states in"="Initialize\n/* some state\n/* another state\nIdle", "error in"=w105) -> ("error out"=w104:errorcluster)  [unwired: 10 in, 2 out]
      }
      frame "Macro: Exit" {
        n32 = call-poly <vilib>:"Polymorphic - Add States(s) To Queue.vi"("queue in"=w111, "states in"="/* some state\n/* another state\nCleanUp\nExit", "error in"=w110) -> ("error out"=w109:errorcluster)  [unwired: 10 in, 2 out]
      }
      frame "------ Action ------" {
      }
      frame "Action: ReadRawDaqQueue" {
        n33 = Unbundle By Name(w117) -> ("RawDaqDataQ"=w115:T19)
        n34 = disable-structure shown="Disabled" {
          disable-tunnel: w115 -> [_ w118 w129]
          frame Enabled {
          }
          frame Disabled {
            n35 = Get Queue Status(queue=w118) -> (queue out=w120:T19, error out=w119:errorcluster, # elements in queue=w121:i32)  [unwired: 2 in, 5 out]
            n36 = case shown="1, Default" w121 {
              selector: w121 -> [_ w124]
              tunnel: w120 -> [_ w123]
              tunnel: w119 -> [_ w122]
              frame 0 {
              }
              frame 1, Default {
                n37 = for {
                  N: w124 -> [_]
                  tunnel: w123 -> [w128]
                  shift-right: [w126] -> _
                  shift-left: w122 -> [w127]
                  tunnel: [w125] -> _ mode=indexing
                  n38 = Dequeue Element(queue=w128, error in (no error)=w127) -> (element=w125:T1, error out=w126:errorcluster)  [unwired: 1 in, 2 out]
                }
              }
            }
          }
          frame Disabled {
            n39 = while {
              tunnel: w129 -> [w134]
              stop <- w133 stop-if-true
              n40 = Dequeue Element(queue=w134, timeout in ms (-1)=5) -> (timed out?=w132:bool, error out=w131:errorcluster)  [unwired: 1 in, 2 out]
              n41 = Compound Arithmetic op=OR(w132, w131) -> (w133:bool)
            }
          }
        }
      }
      frame "Action: Wait" {
        n42 = Scan From String(format string="%d", input string=w137, error in=w136, default 1=u32 0) -> (error out=w135:errorcluster, output 1=w141:u32)  [unwired: 1 in, 2 out]
        n43 = call <userlib>:"Wait (ms)__ogtk.vi"("error in (no error)"=w135, "milliseconds to wait"=w141) -> ("error out"=w139:errorcluster)  [unwired: 8 in, 1 out]
      }
      frame "Action: UpdateSMData" {
        n44 = Match Pattern(string=w150, regular expression=":") -> (before substring=w152:string, after substring=w143:string)  [unwired: 1 in, 2 out]
        n45 = case shown="\"some_data\"" w152 {
          tunnel: w149 -> [_ w159]
          tunnel: w148 -> [_ _]
          tunnel: w147 -> [w153 w158]
          tunnel: [w153 w157] -> w146
          tunnel: w145 -> [w154 w156]
          tunnel: [w154 w155] -> w144
          tunnel: w143 -> [_ _]
          frame Default {
            # "#NOTE:\noptionally add error here."
          }
          frame "some_data" {
            n46 = disable-structure shown="Disabled" {
              disable-tunnel: w159 -> [w166 _]
              disable-tunnel: w156 -> [w164 w167]
              disable-tunnel: [w163 w167] -> w155
              frame Disabled {
                n47 = Variant To Data(error in=w164, type="", Variant=w166) -> (error out=w163:errorcluster)  [unwired: 1 out]
              }
              frame Enabled {
              }
            }
            n48 = disable-structure shown="Disabled" {
              disable-tunnel: w158 -> [w161 w162]
              disable-tunnel: [w160 w162] -> w157
              frame Disabled {
                n49 = Bundle By Name(cluster=w161) -> (w160:T15)  [unwired: 1 in]
              }
              frame Enabled {
              }
            }
          }
        }
      }
    }
  }
  n50 = while {
    shift-right: [w181] -> _
    shift-left: w3 -> [w182]
    shift-right: [w180] -> _
    shift-left: w2 -> [w177]
    shift-right: [w175] -> _
    shift-left: w1 -> [w179]
    shift-right: [w173] -> _
    shift-left: _ -> [w172]
    tunnel: w1 -> [w168]
    stop <- w174 stop-if-true
    # "Data Processing Loop"
    n51 = call <vilib>:"Parse State Queue__JKI_lib_State_Machine.vi"("State Queue"=w179, "Error In (no error)"=w177) -> ("Remaining States"=w176:string, "Current State"=w170:string, "Arguments"=w178:string)  [unwired: 11 in]
    n52 = feedback #1(w168) -> (w169:string)
    n53 = feedback-in #1(w170) -> ()
    n54 = case shown="\"Action: Update ESR Chart Properties\"" w170 {
      tunnel: w182 -> [w186 w191 w198 w200 w218 w226 w234 w395 w401 w407 w412 w416 w456 w480 w489 w508 w522]
      tunnel: [w186 w191 w198 w201 w218 w226 w233 w395 w401 w407 w412 w415 w456 w481 w490 w508 w527] -> w181
      tunnel: w177 -> [w185 w190 w194 w205 w222 w223 w232 w394 w400 w406 w411 w413 w454 w475 w487 w513 w528]
      tunnel: [w185 w190 errorcluster {"status"=FALSE, "code"=0, "source"=""} ("error constant") w205 w222 w223 w231 w394 w400 w406 w411 w414 w455 w476 w488 w513 w536] -> w180
      tunnel: w178 -> [_ _ _ _ _ _ _ _ _ _ _ _ _ _ _ w509 _]
      tunnel: w176 -> [w184 w189 w197 w203 w221 w225 w230 w393 w397 w403 w408 w417 w457 w486 w491 w512 w550]
      tunnel: [w184 w189 w197 w203 w221 w225 w229 w393 w398 w404 w409 w418 w458 w486 w492 w512 w550] -> w175
      tunnel: [_ TRUE _ _ _ _ _ _ _ _ _ _ _ _ _ _ _] -> w174
      tunnel: [w183 w187 w196 w204 w219 w224 w227 w392 w399 w405 w410 w419 w459 w485 w493 w511 w549] -> w173
      tunnel: w172 -> [w183 w187 w196 w204 _ w224 w227 w392 w399 w405 w410 w419 w459 w485 w493 w511 w549]
      tunnel: 10 -> [_ _ _ _ _ _ w228 _ _ _ _ _ _ _ _ _ _]
      tunnel: w169 -> [_ _ w193 _ _ _ _ _ _ _ _ _ _ _ _ _ _]
      frame Default {
      }
      frame "Quit" {
      }
      frame "Error Handler" {
        n55 = call "General Error Handler - show previous state.vi"("error in (no error)"=w194, "Previous State"=w193, "Loop Select"=T33."DataProc Loop - ") -> ()  [unwired: 7 in, 2 out]
      }
      frame "Initialize" {
        n56 = disable-structure shown="Enabled" {
          disable-tunnel: [w208 u32 10 ("upper limit")] -> w202
          disable-tunnel: w200 -> [w206 _]
          frame Disabled {
            n57 = Unbundle By Name(w206) -> ("Measurement config.Samples RMS 9775"=w216:u32, "Measurement config.Data Rate 9775"=w215:dbl)
            n58 = To Double Precision Float(number=w216) -> (double precision float=w213:dbl)
            n59 = To Double Precision Float(number=w215) -> (double precision float=w214:dbl)
            n60 = Divide(x=w213, y=w214) -> (x/y=w212:dbl)
            n61 = expression code="x*1000"(w212) -> (w211:dbl)
            n62 = To Unsigned Long Integer(number=w211) -> (unsigned 32bit integer=w210:u32)
            n63 = In Range and Coerce(upper limit=u32 20000, x=w210, lower limit=u32 20) -> (coerced(x)=w208:u32)  [unwired: 1 out]
          }
          frame Enabled {
          }
        }
        n64 = local write "reset averaging"(TRUE) -> ()
        n65 = Bundle By Name(cluster=w200, "ProcLoopInterval"=w202) -> (w201:T15)
      }
      frame "DE_ Register" {
        n66 = Unbundle By Name(w218) -> ("PrivateAsync Ev"=w220:refnum<user-event>)
        n67 = register-events(w220) -> (reference out=w219:refnum<event-registration>)  [unwired: 2 in, 1 out]
      }
      frame "DE_Unregister" {
        n68 = Unregister For Events(event registration refnum=w224, error in=w223) -> ()  [unwired: 1 out]
      }
      frame "", "EventHandler", "Idle" {
        n69 = event shown="[1] <PrivateAsync Ev>: User Event" {
          selector: w227 -> [_ _]
          dyn-events: _ -> [_ _]
          timeout: w228 -> [_ _]
          tunnel: w234 -> [w237 w268]
          tunnel: [w237 w272] -> w233
          tunnel: w232 -> [w238 w270]
          tunnel: [w239 w271] -> w231
          tunnel: w230 -> [w243 w274]
          tunnel: [w244 w273] -> w229
          event Timeout {
            # "#TODO: maybe add other state\nhandling here."
            n70 = event-data() -> ()  [unwired: 1 in, 1 out]
            n71 = Unbundle By Name(w237) -> ("DAQState"=w241:T23, "ProcessingState"=w240:T14, "ProcLoopInterval"=w236:u32)
            n72 = case shown="\"Running\"" w240 {
              tunnel: [w247 w259] -> w242
              tunnel: w241 -> [w248 w258]
              tunnel: w236 -> [w246 w257]
              tunnel: [w245 w256] -> _
              frame "Idle", Default {
                n73 = case shown="\"Running\"" w248 {
                  tunnel: [_ "Action: FlushDaqQ"] -> w247
                  tunnel: w246 -> [_ w253]
                  tunnel: [u32 100 w250] -> w245
                  frame "Unknown", Default {
                  }
                  frame "Running" {
                    n74 = To Double Precision Float(number=w253) -> (double precision float=w251:dbl)
                    n75 = Multiply(x=w251, y=0.95) -> (x*y=w254:dbl)
                    n76 = To Unsigned Long Integer(number=w254) -> (unsigned 32bit integer=w250:u32)
                  }
                }
              }
              frame "Running" {
                n77 = case shown="\"Running\"" w258 {
                  tunnel: ["" "Action: ProcessDaqData"] -> w259
                  tunnel: w257 -> [_ w263]
                  tunnel: [u32 100 ("ProcLoopInterval") w262] -> w256
                  frame "Unknown", Default {
                  }
                  frame "Running" {
                    n78 = To Double Precision Float(number=w263) -> (double precision float=w264:dbl)
                    n79 = Multiply(x=w264, y=0.95) -> (x*y=w266:dbl)
                    n80 = To Unsigned Long Integer(number=w266) -> (unsigned 32bit integer=w262:u32)
                  }
                }
              }
            }
            n81 = call <userlib>:"Wait (ms)__ogtk.vi"("error in (no error)"=w238, "milliseconds to wait"=u32 10) -> ("error out"=w239:errorcluster)  [unwired: 8 in, 1 out]
            n82 = call <vilib>:"Add State(s) to Queue__JKI_lib_State_Machine.vi"("State(s) in Front (\"\")"=w242, "State(s) in (\"\")"=w243) -> ("States Out"=w244:string)  [unwired: 13 in]
          }
          event User Event {
            n83 = event-data() -> ("vData"=w275:variant, "CmdMsg"=w279:string)  [unwired: 1 in]
            n84 = Scan From String(input string=w279, error in=w270, default 1=PrivateAsynEv_Main--enum."PrivMain.ResetAveraging" ("PrivAsync")) -> (error out=w276:errorcluster, output 1=w277:T34)  [unwired: 2 in, 2 out]
            n85 = case shown="\"PrivMain.CurrInverterUpdated\"" w277 {
              tunnel: w276 -> [w280 w299 w306 w313 w320 w327 w336 w349 w356 w362 w376 w386]
              tunnel: w275 -> [_ w300 w307 w314 w321 w328 w337 _ w357 _ w377 w387]
              tunnel: w268 -> [w282 w297 w305 w312 w319 w326 w335 w348 w354 w363 w373 w384]
              tunnel: [w282 w296 w304 w311 w318 w325 w334 w348 w353 w361 w372 w384] -> w272
              tunnel: [w280 w295 w302 w309 w316 w323 w333 w349 w355 w358 w375 w385] -> w271
              tunnel: ["" _ _ _ _ _ _ "Macro: Exit" _ _ w370 _] -> w269
              tunnel: w268 -> [_ _ _ _ _ _ _ _ _ w367 _ _]
              frame Default {
              }
              frame "PrivMain.UpdateMeasSettings" {
                w298 = T21 {"Data Rate 9775"=3.0, "Data Rate 9215"=1200000.0, "Samples RMS 9215"=480000, "Samples RMS 9775"=3}  # Measurement config
                n86 = Variant To Data(error in=w299, type=w298, Variant=w300) -> (data=w294:T21, error out=w295:errorcluster)
                n87 = Unbundle By Name(w294) -> ("Samples RMS 9215"=w293:u32, "Data Rate 9215"=w284:dbl, "Data Rate 9775"=w283:dbl)
                n88 = local write "Data Rate 9215 (S/s)"(w284) -> ()
                n89 = To Double Precision Float(number=w293) -> (double precision float=w291:dbl)
                n90 = To Double Precision Float(number=w284) -> (double precision float=w292:dbl)
                n91 = local write "Data Rate 9775(S/s)"(w283) -> ()
                n92 = Divide(x=w291, y=w292) -> (x/y=w290:dbl)
                n93 = expression code="x*1000"(w290) -> (w289:dbl)
                n94 = To Unsigned Long Integer(number=w289) -> (unsigned 32bit integer=w288:u32)
                n95 = In Range and Coerce(upper limit=u32 20000, x=w288, lower limit=u32 20) -> (coerced(x)=w286:u32)  [unwired: 1 out]
                n96 = Bundle By Name(cluster=w297, "Measurement config"=w294, "ProcLoopInterval"=w286) -> (w296:T15)
              }
              frame "PrivMain.UpdateAcqMode" {
                w301 = Acquisition_Mode--cluster."3phase"  # Acquisition mode
                n97 = Variant To Data(error in=w306, type=w301, Variant=w307) -> (data=w303:T22, error out=w302:errorcluster)
                n98 = Bundle By Name(cluster=w305, "Acquisition mode"=w303) -> (w304:T15)
              }
              frame "PrivMain.UpdateDAQState" {
                w308 = DAQState--enum."Unknown"  # DAQState
                n99 = Variant To Data(error in=w313, type=w308, Variant=w314) -> (data=w310:T23, error out=w309:errorcluster)
                n100 = Bundle By Name(cluster=w312, "DAQState"=w310) -> (w311:T15)
              }
              frame "PrivMain.UpdateLogState" {
                w315 = LogState--enum."Unknown"  # LogState
                n101 = Variant To Data(error in=w320, type=w315, Variant=w321) -> (data=w317:T24, error out=w316:errorcluster)
                n102 = Bundle By Name(cluster=w319, "LogState"=w317) -> (w318:T15)
              }
              frame "PrivMain.UpdateTDMSState" {
                w322 = TDMSState--enum."Unknown"  # TDMSState
                n103 = Variant To Data(error in=w327, type=w322, Variant=w328) -> (data=w324:T25, error out=w323:errorcluster)
                n104 = Bundle By Name(cluster=w326, "TDMSState"=w324) -> (w325:T15)
              }
              frame "PrivMain.UpdateProcessingState" {
                n105 = Variant To Data(error in=w336, type=cluster{"ProcessingState":T14, variant} {"ProcessingState"=enum."Idle", variant}, Variant=w337) -> (data=w331:cluster{"ProcessingState":T14, variant}, error out=w333:errorcluster)
                n106 = Unbundle(w331) -> ("ProcessingState"=w329:T14, w330:variant)
                n107 = case shown="\"Running\"" w329 {
                  selector: w329 -> [w339 w341]
                  tunnel: w335 -> [w340 w346]
                  tunnel: [w338 w345] -> w334
                  tunnel: w330 -> [_ w344]
                  frame "Idle", Default {
                    # "Update ONLY the state which\nwill disable processing; leave\nthe loop var data alone."
                    n108 = Bundle By Name(cluster=w340, "ProcessingState"=w339) -> (w338:T15)
                  }
                  frame "Running" {
                    w343 = T5 {"DUT ESR avg"=[], "DUT  PF avg"=[], "DUT  Power avg "=[], "DUT processed data"=[], "ESR alarm variables"=[], "Status data"=[], "CurrInverter"=[], "miscellaneous"=[], "DUT INVERTER data"=[]}  # Processing loop variables
                    n109 = Variant To Data(type=w343, Variant=w344) -> (data=w342:T5)  [unwired: 1 in, 1 out]
                    n110 = Bundle By Name(cluster=w346, "ProcessingState"=w341, "Processing loop variables"=w342) -> (w345:T15)
                  }
                }
              }
              frame "PrivMain.Stop&Terminate" {
              }
              frame "PrivMain.CurrInverterUpdated" {
                w351 = T8 {"name"="", "last updated"=timestamp(0 s since 1904-01-01), "type"="", "inverter Info"={"manufacturer"="", "model"="", "product"="", "serial"="", "power class"="", "year manf"=""}, "gain range"={"gain max"=0.0, "gain min"=0.0, "gain increment"=0.0}, "offset range"={"offset max"=0.0, "offset min"=0.0, "offset increment"=0.0}, "gain actual"=0.0, "offset actual"=0.0, "power level"=0.0, "minimum current"=0.0, "resistance single phase"=0.0, "resistance 3 phase"=0.0, "set flag"=0}  # CurrInverter
                n111 = Build Array(w351) -> (w350:T8[])
                n112 = Variant To Data(error in=w356, type=w350, Variant=w357) -> (data=w352:T8[], error out=w355:errorcluster)
                n113 = Bundle By Name(cluster=w354, "Processing loop variables.CurrInverter"=w352) -> (w353:T15)
              }
              frame "PrivMain.UpdateStoreUseESRBaseline" {
                n114 = Unbundle By Name(w367) -> ("Self Reference"=w366:refnum<class "Main.lvclass">)
                n115 = call "Get StoreESR and UseSavedESR Flag reference.vi"("error in (no error)"=w362, "Main in"=w366) -> ("error out"=w358:errorcluster, "UseSavedESR BLine Ref"=w364:refnum<vi>, "StoreESR BLine Ref"=w365:refnum<vi>)  [unwired: 6 in, 1 out]
                n116 = property class="Bool (strict)"(reference=w365) -> ("Visible"=w360:bool)  [unwired: 1 in, 2 out]
                n117 = property class="Bool (strict)"(reference=w364) -> ("Visible"=w359:bool)  [unwired: 1 in, 2 out]
                n118 = Bundle By Name(cluster=w363, "StoreESR BLine Flag"=w360, "UseSavedESR BLine Flag"=w359) -> (w361:T15)
              }
              frame "PrivMain.SetUnsetAlarm&ESRBLine" {
                n119 = Variant To Data(error in=w376, type=FALSE, Variant=w377) -> (data=w368:bool, error out=w375:errorcluster)
                n120 = disable-structure shown="Enabled" {
                  disable-tunnel: w373 -> [w381 w382]
                  disable-tunnel: [w380 w382] -> w372
                  disable-tunnel: w368 -> [w378 _]
                  frame Disabled {
                    n121 = Bundle By Name(cluster=w381, "Alarm on?"=w378, "Inv 1 over threshold?"=FALSE) -> (w380:T15)
                  }
                  frame Enabled {
                  }
                }
                n122 = Select(t="Action: Update Alarm & Baseline", s=w368, f="Action: Unset Alarm") -> (s? t:f=w370:string)
              }
              frame "PrivMain.ResetAveraging" {
                n123 = disable-structure shown="Disabled" {
                  disable-tunnel: w387 -> [w390 _]
                  disable-tunnel: w386 -> [w389 w391]
                  disable-tunnel: [w388 w391] -> w385
                  frame Disabled {
                    n124 = Variant To Data(error in=w389, Variant=w390) -> (error out=w388:errorcluster)  [unwired: 1 in, 1 out]
                  }
                  frame Enabled {
                  }
                }
                n125 = local write "reset averaging"(TRUE) -> ()
              }
            }
            n126 = call <vilib>:"Add State(s) to Queue__JKI_lib_State_Machine.vi"("State(s) in Front (\"\")"=w269, "State(s) in (\"\")"=w274) -> ("States Out"=w273:string)  [unwired: 13 in]
          }
        }
      }
      frame "---------- Macro ----------" {
      }
      frame "Macro: Initialize" {
        n127 = call <vilib>:"Add State(s) to Queue__JKI_lib_State_Machine.vi"("State(s) in Front (\"\")"="Initialize\nDE_ Register", "State(s) in (\"\")"=w397) -> ("States Out"=w398:string)  [unwired: 13 in]
      }
      frame "Macro: Exit" {
        n128 = call <vilib>:"Add State(s) to Queue__JKI_lib_State_Machine.vi"("State(s) in Front (\"\")"="DE_Unregister\nAction: FlushDaqQ >> FlushAll\nQuit", "State(s) in (\"\")"=w403) -> ("States Out"=w404:string)  [unwired: 13 in]
      }
      frame "---------- Action ----------" {
        n129 = call <vilib>:"Add State(s) to Queue__JKI_lib_State_Machine.vi"("State(s) in (\"\")"=w408) -> ("States Out"=w409:string)  [unwired: 14 in]
      }
      frame "Action: Update Alarm & Baseline" {
        n130 = disable-structure shown="Disabled" {
          disable-tunnel: [w437 _] -> w418
          disable-tunnel: w417 -> [w436 _]
          disable-tunnel: w416 -> [w433 _]
          disable-tunnel: [w422 _] -> w415
          disable-tunnel: [w421 _] -> w414
          disable-tunnel: w413 -> [w420 _]
          frame Disabled {
            n131 = Unbundle By Name(w433) -> ("StoreESR BLine Flag"=w432:bool, "StoredESR Baseline"=w431:dbl, "UseSavedESR BLine Flag"=w434:bool, "scaled and averaged raw ESR sum"=w430:dbl)
            n132 = disable-structure shown="Disabled" {
              disable-tunnel: [w441 _] -> w438
              disable-tunnel: w433 -> [w440 _]
              disable-tunnel: [w439 _] -> w424
              frame Disabled {
                n133 = Unbundle By Name(w440) -> ("Alarm on?"=w439:bool, "Self Reference"=w441:refnum<class "Main.lvclass">)
              }
              frame Enabled {
              }
            }
            n134 = call "Get ESR Chart reference.vi"("error in (no error)"=w420, "Main in"=w438) -> ("error out"=w427:errorcluster, "ESR Chart Ref"=w428:refnum<vi>)  [unwired: 7 in, 1 out]
            n135 = property class="WFChart (strict)"(reference=w428, error in=w427) -> (error out=w421:errorcluster, "YScale.Maximum"=w426:dbl)  [unwired: 1 out]
            n136 = Select(t=w431, s=w434, f=w430) -> (s? t:f=w425:dbl)
            n137 = Select(t=w430, s=w432, f=w431) -> (s? t:f=w429:dbl)
            n138 = Bundle By Name(cluster=w433, "StoredESR Baseline"=w429) -> (w423:T15)
            n139 = disable-structure shown="Disabled" {
              disable-tunnel: w426 -> [w446 _]
              disable-tunnel: w425 -> [w445 _]
              disable-tunnel: w424 -> [w444 _]
              disable-tunnel: w423 -> [w443 _]
              disable-tunnel: [w442 _] -> w422
              frame Disabled {
                n140 = case shown="False" w444 {
                  tunnel: w446 -> [_ w453]
                  tunnel: w445 -> [w449 w452]
                  tunnel: w443 -> [w448 w451]
                  tunnel: [w447 w450] -> w442
                  frame True {
                    n141 = Bundle By Name(cluster=w448, "Inv 1 baseline ESR"=w449) -> (w447:T15)
                  }
                  frame False {
                    n142 = Bundle By Name(cluster=w451, "Inv 1 baseline ESR"=w452, "inv 1 esr chart range"=w453) -> (w450:T15)
                  }
                }
              }
              frame Enabled {
              }
            }
            n143 = call <vilib>:"Add State(s) to Queue__JKI_lib_State_Machine.vi"("State(s) in Front (\"\")"="Action: Update ESR Chart Properties\nAction: Reset ESR BLine Flags" ("State(s) in Front (\"\")"), "State(s) in (\"\")"=w436) -> ("States Out"=w437:string)  [unwired: 13 in]
          }
          frame Enabled {
          }
        }
      }
      frame "Action: Update ESR Chart Properties" {
        n144 = disable-structure shown="Disabled" {
          disable-tunnel: w456 -> [w468 _]
          disable-tunnel: [w461 _] -> w455
          disable-tunnel: w454 -> [w460 _]
          frame Disabled {
            n145 = Unbundle By Name(w468) -> ("StoredESR Baseline"=w472:dbl, "UseSavedESR BLine Flag"=w473:bool, "scaled and averaged raw ESR sum"=w471:dbl)
            n146 = Unbundle By Name(w468) -> ("Self Reference"=w474:refnum<class "Main.lvclass">)
            n147 = call "Get ESR Chart reference.vi"("error in (no error)"=w460, "Main in"=w474) -> ("error out"=w469:errorcluster, "ESR Chart Ref"=w470:refnum<vi>)  [unwired: 7 in, 1 out]
            n148 = Select(t=w472, s=w473, f=w471) -> (s? t:f=w467:dbl)
            n149 = Multiply(x=w467, y=4.0) -> (x*y=w465:dbl)
            n150 = property class="WFChart (strict)"(reference=w470, error in=w469, "YScale.FormatString"="%.3e", "YScale.Maximum"=w465, "YScale.Minimum"=0.0 ("Y Scale.Range:Minimum"), "History Data"=T35 []) -> (error out=w461:errorcluster)  [unwired: 1 out]
          }
          frame Enabled {
          }
        }
        n151 = call <vilib>:"Add State(s) to Queue__JKI_lib_State_Machine.vi"("State(s) in (\"\")"=w457) -> ("States Out"=w458:string)  [unwired: 14 in]
      }
      frame "Action: Reset ESR BLine Flags" {
        w477 = FALSE ("Value")
        n152 = Unbundle By Name(w480) -> ("Self Reference"=w482:refnum<class "Main.lvclass">)
        n153 = call "Get StoreESR and UseSavedESR Flag reference.vi"("error in (no error)"=w475, "Main in"=w482) -> ("error out"=w479:errorcluster, "UseSavedESR BLine Ref"=w483:refnum<vi>, "StoreESR BLine Ref"=w484:refnum<vi>)  [unwired: 6 in, 1 out]
        n154 = property class="Bool (strict)"(reference=w483, error in=w479, "Value"=w477) -> (error out=w478:errorcluster)  [unwired: 1 out]
        n155 = property class="Bool (strict)"(reference=w484, error in=w478, "Value"=w477) -> (error out=w476:errorcluster)  [unwired: 1 out]
        n156 = Bundle By Name(cluster=w480, "StoreESR BLine Flag"=w477, "UseSavedESR BLine Flag"=w477) -> (w481:T15)
      }
      frame "Action: Unset Alarm" {
        n157 = disable-structure shown="Disabled" {
          disable-tunnel: [w498 w506] -> w490
          disable-tunnel: w489 -> [w497 w506]
          disable-tunnel: [w496 _] -> w488
          disable-tunnel: w487 -> [w495 _]
          frame Disabled {
            w494 = FALSE
            n158 = Unbundle By Name(w497) -> ("inv 1 esr chart range"=w499:dbl)
            n159 = Unbundle By Name(w497) -> ("Self Reference"=w505:refnum<class "Main.lvclass">)
            n160 = call "Get ESR Chart reference.vi"("error in (no error)"=w495, "Main in"=w505) -> ("error out"=w503:errorcluster, "ESR Chart Ref"=w504:refnum<vi>)  [unwired: 7 in, 1 out]
            n161 = property class="WFChart (strict)"(reference=w504, error in=w503, "YScale.FormatString"="%#_g", "YScale.Maximum"=w499, "YScale.Minimum"=0.0 ("Y Scale.Range:Minimum"), "History Data"=T35 []) -> (error out=w496:errorcluster)  [unwired: 1 out]
            n162 = Bundle By Name(cluster=w497, "Alarm on?"=w494, "Inv 1 over threshold?"=w494) -> (w498:T15)
          }
          frame Enabled {
          }
        }
        n163 = call <vilib>:"Add State(s) to Queue__JKI_lib_State_Machine.vi"("State(s) in (\"\")"=w491) -> ("States Out"=w492:string)  [unwired: 14 in]
      }
      frame "Action: FlushDaqQ" {
        n164 = Unbundle By Name(w508) -> ("RawDaqDataQ"=w510:T19)
        n165 = Flush Queue(queue=w510) -> (error out=w507:errorcluster)  [unwired: 1 in, 2 out]
        n166 = case shown="\"FlushAll\"" w509 {
          tunnel: w508 -> [_ w517]
          tunnel: w507 -> [_ _]
          frame "False", Default {
          }
          frame "FlushAll" {
            n167 = Unbundle By Name(w517) -> ("InverterWaveformsQ"=w514:T20, "InvWfmsQ-DT"=w515:T20, "DPAuxDataQ"=w516:T26)
            n168 = Flush Queue(queue=w516) -> ()  [unwired: 1 in, 3 out]
            n169 = Flush Queue(queue=w515) -> ()  [unwired: 1 in, 3 out]
            n170 = Flush Queue(queue=w514) -> ()  [unwired: 1 in, 3 out]
          }
        }
      }
      frame "Action: ProcessDaqData" {
        n171 = Unbundle By Name(w522) -> ("InvWfmsQ-DT"=w537:T20, "DPAuxDataQ"=w538:T26, "InverterWaveformsQ"=w539:T20)
        n172 = Unbundle By Name(w522) -> ("TDMSState"=w541:T25)
        n173 = Unbundle By Name(w522) -> ("Acquisition mode"=w520:T22, "Processing loop variables"=w546:T5, "RawDaqDataQ"=w519:T19)
        n174 = Unbundle By Name(w522) -> ("LogState"=w523:T24)
        n175 = Not Equal?(x=w541, y=TDMSState--enum."Running") -> (x != y?=w534:bool)
        n176 = Not Equal?(x=w523, y=LogState--enum."Running") -> (x != y?=w521:bool)
        n177 = Get Queue Status(queue=w519, error in (no error)=w528) -> (queue out=w532:T19, error out=w529:errorcluster, # elements in queue=→"RawDaqDataQ size":i32)  [unwired: 1 in, 5 out]
        n178 = Dequeue Element(queue=w532, timeout in ms (-1)=8000, error in (no error)=w529) -> (element=w547:T1, timed out?=w531:bool, error out=w548:errorcluster)  [unwired: 1 out]
        n179 = case shown="False" w531 {
          tunnel: w548 -> [w568 w585]
          tunnel: w547 -> [w563 _]
          tunnel: w546 -> [w565 w584]
          tunnel: "Data Rate 9215 (S/s)" -> [w566 _]
          tunnel: "ESR scaling" -> [w552 _]
          tunnel: "UseDummyVrms" -> [w562 _]
          tunnel: "Dummy Vrms" -> [w561 _]
          tunnel: "reset averaging" -> [w555 _]
          tunnel: w539 -> [w575 _]
          tunnel: w538 -> [w574 _]
          tunnel: w537 -> [w572 _]
          tunnel: [w570 w585] -> w536
          tunnel: "Settings.Signal scaling" -> [w564 _]
          tunnel: w534 -> [w558 _]
          tunnel: [w557 w584] -> w526
          tunnel: w521 -> [w556 _]
          tunnel: w520 -> [w554 _]
          tunnel: "Data Rate 9775(S/s)" -> [w553 _]
          frame False {
            w578 = FALSE  # UpdateTS (T)
            n180 = call "Process DAQ Data.vi"("reset averaging"=w555, "Processing loop variables"=w565, "Data Rate 9775(S/s)"=w553, "RawDAQData in"=w563, "Signal scaling"=w564, "error in"=w568, "Data Rate 9215 (S/s)"=w566, "ESR scaling"=w552, "Acquisition mode"=w554, "Use dummy Vout?"=w562, "Dummy Vrms"=w561) -> ("InverterWaveforms"=w559:T12, "Processing loop vars out"=w557:T5, "DataProcAuxData"=w551:T36[], "MeasData"=w560:T37, "error out"=w567:errorcluster)  [unwired: 4 in]
            n181 = case shown="False" w558 {
              tunnel: w575 -> [w582 _]
              tunnel: [w581 errorcluster {"status"=FALSE, "code"=0, "source"=""} ("error constant")] -> w573
              tunnel: w559 -> [w580 _]
              frame False {
                n182 = Enqueue Element(queue=w582, element=w580) -> (error out=w581:errorcluster)  [unwired: 2 in, 2 out]
              }
              frame True {
              }
            }
            n183 = case shown="True" w555 {
              frame False {
              }
              frame True {
                n184 = local write "reset averaging"(FALSE) -> ()
              }
            }
            n185 = call "Set MeasData in Q.vi"("UpdateTS (T)"=w578, "error in (no error)"=w567, "MeasData out"=w560) -> ("error out"=w577:errorcluster)  [unwired: 7 in, 1 out]
            n186 = Enqueue Element(queue=w574, element=w551, error in (no error)=w573) -> (error out=w571:errorcluster)  [unwired: 1 in, 2 out]
            n187 = call "Get MeasData Q and Insert Logging Data.vi"("error in"=w577, "bypass"=w556) -> ("error out"=w576:errorcluster)  [unwired: 6 in, 2 out]
            n188 = Enqueue Element(queue=w572, element=w559, error in (no error)=w571) -> (error out=w569:errorcluster)  [unwired: 1 in, 2 out]
            n189 = Merge Errors(w569, w576) -> (w570:errorcluster)
            "DAQ data" <- w563
          }
          frame True {
          }
        }
        n190 = Bundle By Name(cluster=w522, "Processing loop variables"=w526) -> (w527:T15)
      }
    }
  }
  n191 = while {
    shift-right: [w596] -> _
    shift-left: w3 -> [w595]
    shift-right: [w599] -> w6
    shift-left: w2 -> [w594]
    shift-right: [w598] -> _
    shift-left: w10 -> [w600]
    shift-right: [w593] -> _
    shift-left: _ -> [w592]
    tunnel: w9 -> [w590]
    tunnel: w8 -> [w589]
    tunnel: w4 -> [w588]
    stop <- w597 stop-if-true
    n192 = call <vilib>:"Parse State Queue__JKI_lib_State_Machine.vi"("State Queue"=w600, "Error In (no error)"=w594) -> ("Remaining States"=w602:string, "Current State"=w587:string, "Arguments"=w601:string)  [unwired: 11 in]
    n193 = feedback #2(w588) -> (w586:string)
    n194 = feedback-in #2(w587) -> ()
    n195 = case shown="\"\", \"Event Structure\", \"Idle\"" w587 {
      selector: w587 -> [w604 _ _ _ _ _ _ _ _ _ _ _ _ _ _ _ _ _ _ _ _ _ _ _]
      tunnel: w602 -> [w608 w623 w629 w637 w818 w831 w839 w853 w857 w862 w876 w883 w888 w896 w905 w917 w944 w950 w961 w966 w977 w1015 w1026 w1040]
      tunnel: w601 -> [_ _ _ _ _ _ _ _ _ _ _ _ _ _ w900 w911 _ _ _ _ _ _ w1016 _]
      tunnel: w595 -> [w606 w620 w627 w635 w815 w822 w836 w850 w856 w859 w867 w878 w885 w891 w903 w913 w941 w947 w958 w963 w973 w1011 w1024 w1033]
      tunnel: [w610 errorcluster {"status"=FALSE, "code"=0, "source"=""} ("error out") w626 w634 w816 w828 w832 w851 w854 w860 w874 w879 w886 w892 w901 w914 w942 w948 w959 w964 w968 w997 w1017 w1028] -> w599
      tunnel: w594 -> [w609 w619 w626 w633 w816 w828 w833 w844 w854 w860 w874 w880 w886 w893 w902 w915 w942 w948 w959 w964 w967 w996 w1018 w1034]
      tunnel: [w607 w622 w628 w636 w817 w830 w838 w853 w857 w861 w875 w882 w887 w895 w904 w916 w943 w949 w960 w965 w976 w1014 w1025 w1039] -> w598
      tunnel: [_ _ TRUE _ _ _ _ _ _ _ _ _ _ _ _ _ _ _ _ _ _ _ _ _] -> w597
      tunnel: [w606 w620 w627 w632 w815 w829 w836 w850 w856 w859 w870 w878 w885 w891 w903 w913 w941 w947 w958 w963 w973 w1011 w1024 w1033] -> w596
      tunnel: [w603 w617 w624 w630 w814 w819 w837 w852 w855 w858 w869 w877 w884 w894 w899 w910 w940 w946 w952 w962 w975 w1013 w1023 w1038] -> w593
      tunnel: w592 -> [w603 w617 w624 w630 w814 w819 w837 _ w855 w858 w869 w877 w884 w894 w899 w910 w940 w946 w952 w962 w975 w1013 w1023 w1038]
      tunnel: 200 ("Timeout") -> [_ _ _ w631 _ _ _ _ _ _ _ _ _ _ _ _ _ _ _ _ _ _ _ _]
      tunnel: w590 -> [_ _ _ _ _ _ _ _ _ _ _ _ _ _ _ _ _ w945 _ _ _ _ _ _]
      tunnel: w589 -> [_ _ _ _ _ _ _ _ _ _ _ _ _ _ _ _ _ _ w951 _ _ _ _ _]
      tunnel: w586 -> [_ w616 _ _ _ _ _ _ _ _ _ _ _ _ _ _ _ _ _ _ _ _ _ _]
      frame Default {
        w613 = 42 items=["No error", "Argument error", "Memory is full", "Out of zone", "End of file", "File already open", "Generic file I/O error", "File not found", "File permission error", "Disk is full", "Duplicate path", "Too many files open", "System feature not enabled", "Resource file not found", "Cannot add resource", "Resource not found", "Image not found", "Image memory error", "Pen does not exist", "Config type invalid", "Config token not found", "Config parse error", "Config memory error", "Bad external code format", "Bad external code offset", "External code not present", "Null window", "Destroy window error", "Null menu", "Print aborted", "Bad print record", "Print driver error", "Windows error during printing", "Memory error during printing", "Print dialog error", "Generic print error", "Invalid device refnum", "Device not found", "Device parameter error", "Device unit error", "Cannot open device", "Device call aborted", "Generic error", "Cancelled by user", "Object ID too low", "Object ID too high", "Object not in heap", "Unknown heap", "Unknown object (invalid DefProc)", "Unknown object (DefProc not in table)", "Message out of range", "Invalid (null) method", "Unknown message", "Manager call not supported", "Bad address", "Network operation in progress", "Network operation timed out", "Connection is busy", "Network attribute not supported", "Network error", "Address in use", "System out of memory", "Connection aborted", "Connection refused", "Not connected", "Already connected", "Connection closed", "Initialization error (interapplication manager)", "Bad occurrence", "Wait on unbound occurrence handler", "Occurrence queue overflow", "Datalog type conflict", "Unused", "Unrecognized type (interapplication manager)", "Memory corrupt", "Failed to make temporary DLL", "Old CIN version", "Drag socket not found", "Failed to load drop-object", "Failed to register OLE object", "Failed to release OLE object", "Format specifier type mismatch", "Unknown format specifier", "Too few format specifiers", "Too many format specifiers", "Scan failed", "Newer CIN version", "Error converting to variant", "Runtime menu error", "Password tampered", "Variant attribute not found", "Incompatible variant data type", "Event data is not available", "Event Store is not present", "Occurrence is not found", "Event Queue is not created", "Event info is not available", "Refnum passed is NULL", "Error retrieving Class GUID", "Error retrieving CoClass GUID", "Error retrieving TypeLib GUID.", "Bad built application magic bytes.", "Specific driver is different from the specific driver associated with the Logical Name.", "There is no session opened to the class driver.", "Max Error", "MAX - Error with config objects", "MAX - Error loading configuration", "MAX - Group not supported"]
        # "Current State"
        n196 = Format Into String(format string="Software Exception: Unhandled State \"%s\"." ("message"), error in=w609, w604) -> (resulting string=w612:string, error out=w611:errorcluster)  [unwired: 1 in]
        n197 = call <vilib>:"Error Cluster From Error Code.vi"("show call chain? (False)"=TRUE, "error in (no error)"=w611, "error message (\"\")"=w612, "error code (0)"=w613) -> ("error out"=w610:errorcluster)  [unwired: 5 in]
        n198 = call <vilib>:"Add State(s) to Queue__JKI_lib_State_Machine.vi"("State(s) in (\"\")"=w608) -> ("States Out"=w607:string)  [unwired: 14 in]
      }
      frame "Error Handler" {
        n199 = call "General Error Handler - show previous state.vi"("error in (no error)"=w619, "Previous State"=w616, "Loop Select"=enum16{"Event Loop -", "Async Loop -"}."Event Loop -") -> ()  [unwired: 7 in, 2 out]
        n200 = call <vilib>:"Add State(s) to Queue__JKI_lib_State_Machine.vi"("State(s) in Front (\"\")"="/* Post Error States", "State(s) in (\"\")"=w623) -> ("States Out"=w622:string)  [unwired: 13 in]
      }
      frame "Exit" {
        n201 = call <vilib>:"Add State(s) to Queue__JKI_lib_State_Machine.vi"("State(s) in (\"\")"=w629) -> ("States Out"=w628:string)  [unwired: 14 in]
      }
      frame "", "Event Structure", "Idle" {
        n202 = event shown="[10] <Public Events.UpdateControlValue Ev>: User Event" {
          selector: w630 -> [_ _ _ _ _ _ _ _ _ _ _ _ _]
          dyn-events: _ -> [_ _ _ _ _ _ _ _ _ _ _ _ _]
          timeout: w631 -> [_ _ _ _ _ _ _ _ _ _ _ _ _]
          tunnel: w637 -> [w641 w646 w652 w655 w662 w678 w731 w749 w757 w766 w772 w804 w813]
          tunnel: [w640 w645 w651 w654 w661 w677 w731 w749 w757 w766 w772 w804 w813] -> w636
          tunnel: w635 -> [w638 w643 w649 w657 w665 w667 w722 w744 w752 w760 w771 w799 w808]
          tunnel: [w639 w644 w650 w658 w666 w675 w724 w747 w755 w764 w767 w802 w811] -> w634
          tunnel: w633 -> [w639 w644 w650 w658 w666 w674 w723 w746 w754 w763 w768 w801 w810]
          tunnel: [w638 w643 w649 w657 w664 w669 w725 w745 w753 w762 w771 w800 w809] -> w632
          event Timeout {
            n203 = event-data() -> ()  [unwired: 1 in, 1 out]
            n204 = call <vilib>:"Add State(s) to Queue__JKI_lib_State_Machine.vi"("State(s) in (\"\")"=w641) -> ("States Out"=w640:string)  [unwired: 14 in]
          }
          event "Exit": Value Change {
            n205 = event-data() -> ()  [unwired: 1 in, 1 out]
            n206 = call <vilib>:"Add State(s) to Queue__JKI_lib_State_Machine.vi"("State(s) in Front (\"\")"="Macro: Exit", "State(s) in (\"\")"=w646) -> ("States Out"=w645:string)  [unwired: 13 in]
          }
          event Panel Close? {
            n207 = event-data() -> ()  [unwired: 1 in, 1 out]
            n208 = event-data("Discard?"=TRUE) -> ()  [unwired: 1 in, 1 out]
            n209 = call <vilib>:"Add State(s) to Queue__JKI_lib_State_Machine.vi"("State(s) in Front (\"\")"="Macro: Exit", "State(s) in (\"\")"=w652) -> ("States Out"=w651:string)  [unwired: 13 in]
          }
          event Menu Selection (User) {
            n210 = event-data() -> ("ItemTag"=w656:string)  [unwired: 1 in, 2 out]
            n211 = case shown="\"False\", Default" w656 {
              tunnel: [""] -> w653
              frame "False", Default {
              }
            }
            n212 = call <vilib>:"Add State(s) to Queue__JKI_lib_State_Machine.vi"("State(s) in Front (\"\")"=w653, "State(s) in (\"\")"=w655) -> ("States Out"=w654:string)  [unwired: 13 in]
          }
          event User Event {
            n213 = event-data() -> ("notifier out"=w663:refnum<notifier>)  [unwired: 1 in]
            n214 = Bundle By Name(cluster=w665, "process sync"=w663) -> (w664:T15)
            n215 = call <vilib>:"Add State(s) to Queue__JKI_lib_State_Machine.vi"("State(s) in Front (\"\")"="Macro: Exit", "State(s) in (\"\")"=w662) -> ("States Out"=w661:string)  [unwired: 13 in]
          }
          event User Event {
            n216 = event-data() -> ("CmdMsg"=w672:string, "vData"=w676:variant)  [unwired: 1 in, 1 out]
            n217 = Unbundle By Name(w667) -> ("Self Reference"=w668:refnum<class "Main.lvclass">)
            n218 = call "get async cmd.vi"("error in (no error)"=w674, "Cmd String in"=w672) -> ("error out"=w673:errorcluster, "AsyncCmd"=w671:T43)  [unwired: 8 in]
            n219 = case shown="\"Main.StopProcessing\"" w671 {
              tunnel: w676 -> [_ _ w694 w707]
              tunnel: w673 -> [w684 w686 w688 w715]
              tunnel: [w683 w686 w695 w708] -> w675
              tunnel: [_ _ "Action: StartProcessing" "Action: StopProcessing"] -> w670
              tunnel: w667 -> [w679 w685 w698 w713]
              tunnel: [w679 w685 w697 w712] -> w669
              tunnel: w668 -> [_ _ w690 w711]
              tunnel: w667 -> [_ _ _ _]
              frame Default {
                n220 = call <vilib>:"Build Error Cluster_ModKT .vi"("Prepend String (\"\")"="Invalid Async Cmd" ("Prepend String (\"\")"), "code"=42, "error? (F)"=TRUE, "error in (no error)"=w684) -> ("error out"=w683:errorcluster)  [unwired: 3 in, 1 out]
              }
              frame "Main.RefreshInverterList" {
              }
              frame "Main.StartProcessing" {
                w693 = T44 {"InverterInfo"={"Inverter ID"=""}, "ProcessInitParams"={"MinCurrThreshold"=1.5, "NumPF RdsToAvg"=10, "ESR alarm threshhold (%)"=200.0, "# readings to average"=40}}  # StartProcInitParams
                w696 = ProcessingState--enum."Running" ("ProcessingState")
                n221 = disable-structure shown="Enabled" {
                  disable-tunnel: w688 -> [w704 w706]
                  disable-tunnel: [w703 w706] -> _
                  disable-tunnel: w694 -> [w702 _]
                  disable-tunnel: w693 -> [w701 w705]
                  disable-tunnel: [w700 w705] -> w692
                  frame Enabled {
                    n222 = Variant To Data(error in=w704, type=w701, Variant=w702) -> (data=w700:T44, error out=w703:errorcluster)
                  }
                  frame Disabled {
                  }
                }
                n223 = Unbundle(w692) -> ("InverterInfo"=w689:T27)  [unwired: 1 out]
                n224 = property class="Main.lvclass"(reference=w690, error in=w688, "Accessors:InverterInfo*"=w689) -> (reference out=w691:refnum<class "Main.lvclass">, error out=w687:errorcluster)
                n225 = Bundle By Name(cluster=w698, "ProcessingState"=w696, "vData"=w694) -> (w697:T15)
                n226 = call "Fire ProcessingStateChanged Event_DAQ.vi"("error in (no error)"=w687, "DAQState"=w696, "Main in"=w691) -> ("error out"=w695:errorcluster)  [unwired: 7 in, 1 out]
              }
              frame "Main.StopProcessing" {
                w710 = ProcessingState--enum."Idle" ("ProcessingState")
                n227 = disable-structure shown="Enabled" {
                  disable-tunnel: w715 -> [w719 w721]
                  disable-tunnel: [w718 w721] -> w709
                  disable-tunnel: w707 -> [w717 w720]
                  disable-tunnel: [w716 w720] -> _
                  frame Disabled {
                    n228 = Variant To Data(error in=w719, Variant=w717) -> (data=w716:variant, error out=w718:errorcluster)  [unwired: 1 in]
                  }
                  frame Enabled {
                  }
                }
                n229 = call "Fire ProcessingStateChanged Event_DAQ.vi"("error in (no error)"=w709, "DAQState"=w710, "Main in"=w711) -> ("error out"=w708:errorcluster)  [unwired: 7 in, 1 out]
                n230 = Bundle By Name(cluster=w713, "ProcessingState"=w710, "vData"=w707) -> (w712:T15)
              }
            }
            n231 = call <vilib>:"Add State(s) to Queue__JKI_lib_State_Machine.vi"("State(s) in Front (\"\")"=w670, "State(s) in (\"\")"=w678) -> ("States Out"=w677:string)  [unwired: 13 in]
          }
          event User Event {
            n232 = event-data() -> ("CmdMsg"=w730:string, "vData"=w726:variant)  [unwired: 1 in, 1 out]
            n233 = Unbundle By Name(w722) -> ("Self Reference"=w729:refnum<class "Main.lvclass">)
            n234 = call "get async msg.vi"("error in (no error)"=w723, "Msg String in"=w730) -> ("error out"=w727:errorcluster, "AsyncMsg"=w728:T46)  [unwired: 8 in]
            n235 = case shown="\"Main.CurrInverterUpdated\"" w728 {
              tunnel: w729 -> [_ _]
              tunnel: w727 -> [w733 w739]
              tunnel: w726 -> [_ w740]
              tunnel: [w733 w738] -> w724
              tunnel: w722 -> [w732 w737]
              tunnel: [w732 w736] -> w725
              tunnel: w722 -> [_ _]
              frame Default {
              }
              frame "Main.CurrInverterUpdated" {
                n236 = Variant To Data(error in=w739, type=T8[] [], Variant=w740) -> (data=w735:T8[], error out=w738:errorcluster)
                n237 = Bundle By Name(cluster=w737, "Processing loop variables.CurrInverter"=w735) -> (w736:T15)
              }
            }
          }
          event User Event {
            n238 = event-data() -> ("NEW Settings"=w741:T47)  [unwired: 1 in, 6 out]
            n239 = Unbundle By Name(w744) -> ("Self Reference"=w743:refnum<class "Main.lvclass">)
            n240 = Unbundle By Name(w741) -> ("Measurement config"=w742:T21)
            n241 = call "Fire Private Event.vi"("error in (no error)"=w746, "vData"=w742, "PrivAsync"=PrivateAsynEv_Main--enum."PrivMain.UpdateMeasSettings", "Main in"=w743) -> ("error out"=w747:errorcluster)  [unwired: 6 in, 1 out]
            n242 = Bundle By Name(cluster=w744, "Measurement config"=w742) -> (w745:T15)
          }
          event User Event {
            n243 = event-data() -> ("NEW AcqMode"=w750:T22)  [unwired: 1 in, 6 out]
            n244 = Unbundle By Name(w752) -> ("Self Reference"=w751:refnum<class "Main.lvclass">)
            n245 = call "Fire Private Event.vi"("error in (no error)"=w754, "vData"=w750, "PrivAsync"=PrivateAsynEv_Main--enum."PrivMain.UpdateAcqMode", "Main in"=w751) -> ("error out"=w755:errorcluster)  [unwired: 6 in, 1 out]
            n246 = Bundle By Name(cluster=w752, "Acquisition mode"=w750) -> (w753:T15)
          }
          event User Event {
            n247 = event-data() -> ("NEW State"=w758:T30)  [unwired: 1 in, 6 out]
            n248 = Unbundle By Name(w760) -> ("Self Reference"=w759:refnum<class "Main.lvclass">)
            n249 = Unbundle By Name(w758) -> ("DAQState"=w761:T23)
            n250 = call "Fire Private Event.vi"("error in (no error)"=w763, "vData"=w761, "PrivAsync"=PrivateAsynEv_Main--enum."PrivMain.UpdateDAQState", "Main in"=w759) -> ("error out"=w764:errorcluster)  [unwired: 6 in, 1 out]
            n251 = Bundle By Name(cluster=w760, "DAQState"=w761) -> (w762:T15)
          }
          event User Event {
            n252 = event-data() -> ("ControlLabel"=w770:string, "vData"=w769:variant)  [unwired: 1 in, 1 out]
            n253 = case shown="\"ESR scaling\"" w770 {
              tunnel: w769 -> [_ w779 w784 w789 w795]
              tunnel: w768 -> [w773 w776 w782 w787 w793]
              tunnel: [w773 w775 w781 w786 w792] -> w767
              frame "False", Default {
              }
              frame "ESR scaling" {
                n254 = Build Array(T3 {"Gain"=0.0, "Offset"=0.0} ("ESR scaling")) -> (w774:T3[])
                n255 = Variant To Data(error in=w776, type=w774, Variant=w779) -> (data=w777:T3[], error out=w775:errorcluster)
                n256 = local write "ESR scaling"(w777) -> ()
              }
              frame "UseDummyVrms" {
                n257 = Variant To Data(error in=w782, type=FALSE, Variant=w784) -> (data=w783:bool, error out=w781:errorcluster)
                n258 = local write "UseDummyVrms"(w783) -> ()
              }
              frame "Dummy Vrms" {
                n259 = Variant To Data(error in=w787, type=0.0, Variant=w789) -> (data=w788:dbl, error out=w786:errorcluster)
                n260 = local write "Dummy Vrms"(w788) -> ()
              }
              frame "Signal scaling" {
                n261 = Build Array(T4 {"Iin ripple gain"=13.333, "Iout ripple gain"=13.333, "Iout 60Hz gain "=14.286, "Vout 60Hz gain "=20.0, "Iin ripple offest"=0.0, "Iout ripple offset"=0.0, "Iout 60Hz offset"=0.0, "Vout 60Hz offset"=0.0} ("Signal scaling")) -> (w790:T4[])
                n262 = Variant To Data(error in=w793, type=w790, Variant=w795) -> (data=w794:T4[], error out=w792:errorcluster)
                n263 = local write "Settings.Signal scaling"(w794) -> ()
              }
            }
          }
          event User Event {
            n264 = event-data() -> ("NEW State"=w796:T48)  [unwired: 1 in, 6 out]
            n265 = Unbundle By Name(w799) -> ("Self Reference"=w798:refnum<class "Main.lvclass">)
            n266 = Unbundle By Name(w796) -> ("LogState"=w797:T24)
            n267 = call "Fire Private Event.vi"("error in (no error)"=w801, "vData"=w797, "PrivAsync"=PrivateAsynEv_Main--enum."PrivMain.UpdateLogState", "Main in"=w798) -> ("error out"=w802:errorcluster)  [unwired: 6 in, 1 out]
            n268 = Bundle By Name(cluster=w799, "LogState"=w797) -> (w800:T15)
          }
          event User Event {
            n269 = event-data() -> ("NEW State"=w806:T49)  [unwired: 1 in]
            n270 = Unbundle By Name(w808) -> ("Self Reference"=w807:refnum<class "Main.lvclass">)
            n271 = Unbundle By Name(w806) -> ("TDMSState"=w805:T25)
            n272 = call "Fire Private Event.vi"("error in (no error)"=w810, "vData"=w805, "PrivAsync"=PrivateAsynEv_Main--enum."PrivMain.UpdateTDMSState", "Main in"=w807) -> ("error out"=w811:errorcluster)  [unwired: 6 in, 1 out]
            n273 = Bundle By Name(cluster=w808, "TDMSState"=w805) -> (w809:T15)
          }
        }
      }
      frame "---------- Core ----------" {
        n274 = call <vilib>:"Add State(s) to Queue__JKI_lib_State_Machine.vi"("State(s) in (\"\")"=w818) -> ("States Out"=w817:string)  [unwired: 14 in]
      }
      frame "Initialize Core Data" {
        # "originally closed?"
        # "exe?"
        n275 = property class="VI"() -> ("Front Panel.Open"=w827:bool)  [unwired: 2 in, 2 out]
        n276 = property class="App"() -> ("App.Kind"=w826:T39)  [unwired: 2 in, 2 out]
        n277 = control-ref of="Current VI Reference"() -> (w820:refnum<vi>)
        n278 = Not(x=w827) -> (.not. x?=w824:bool)
        n279 = Equal?(x=w826, y=T39."Run Time System" ("Application:Kind")) -> (x = y?=w823:bool)
        n280 = Or(x=w824, y=w823) -> (x .or. y?=w821:bool)
        n281 = Bundle By Name(cluster=w822, "Core.Current VI Reference"=w820, "Core.Close Panel on Exit?"=w821) -> (w829:T15)
        n282 = call <vilib>:"Add State(s) to Queue__JKI_lib_State_Machine.vi"("State(s) in (\"\")"=w831) -> ("States Out"=w830:string)  [unwired: 14 in]
      }
      frame "Process Sync" {
        n283 = Unbundle By Name(w836) -> ("process sync"=w835:refnum<notifier>)
        n284 = Send Notification(notification=TRUE, notifier=w835, error in (no error)=w833) -> (error out=w832:errorcluster)  [unwired: 1 out]
        n285 = call <vilib>:"Add State(s) to Queue__JKI_lib_State_Machine.vi"("State(s) in (\"\")"=w839) -> ("States Out"=w838:string)  [unwired: 14 in]
      }
      frame "DE_Register" {
        n286 = Unbundle By Name(w850) -> ("Public Events"=w849:T18, "PrivateAsync Ev"=w846:refnum<user-event>, "Dependency.DAQ"=w848:refnum<class "DAQ_Engine.lvclass">, "Dependency.Log_Engine"=w845:refnum<class "Log_Engine.lvclass">)
        n287 = property class="DAQ_Engine.lvclass"(reference=w848, error in=w844) -> (error out=w841:errorcluster, "Accessors:PublicEvents*"=w847:T50)  [unwired: 1 out]
        n288 = property class="Log_Engine.lvclass"(reference=w845, error in=w844) -> (error out=w842:errorcluster, "Accessors:PublicEvents*"=w843:T51)  [unwired: 1 out]
        n289 = Merge Errors(w841, w842) -> (w840:errorcluster)
        n290 = register-events(error in=w840, w849, w847, w846, w843) -> (reference out=w852:refnum<event-registration>, error out=w851:errorcluster)  [unwired: 1 in]
      }
      frame "DE_Unregister" {
        n291 = Unregister For Events(event registration refnum=w855, error in=w854) -> ()  [unwired: 1 out]
      }
      frame "---------- Data ----------" {
        n292 = call <vilib>:"Add State(s) to Queue__JKI_lib_State_Machine.vi"("State(s) in (\"\")"=w862) -> ("States Out"=w861:string)  [unwired: 14 in]
      }
      frame "Data: Initialize" {
        w871 = T52 {"Current VI Reference"=refnum, "Close Panel on Exit?"=FALSE}  # Core
        w873 = TRUE  # Your Boolean data
        w872 = ""  # Your string data
        # "#NOTE: possibly get this from Main UI instead."
        n293 = Unbundle By Name(w867) -> ("Settings.Signal scaling"=w868:T4[])
        n294 = Unbundle By Name(w867) -> ("Dependency.DAQ"=w866:refnum<class "DAQ_Engine.lvclass">)
        n295 = local write "Settings.Signal scaling"(w868) -> ()
        n296 = property class="DAQ_Engine.lvclass"(reference=w866) -> ("Accessors:MeasSettings*"=w865:T21)  [unwired: 1 in, 2 out]
        n297 = Unbundle By Name(w865) -> ("Data Rate 9215"=w864:dbl, "Data Rate 9775"=w863:dbl)
        n298 = local write "Data Rate 9775(S/s)"(w863) -> ()
        n299 = local write "Data Rate 9215 (S/s)"(w864) -> ()
        n300 = Bundle By Name(cluster=w867, "Core"=w871, "Your Boolean data"=w873, "Your string data"=w872) -> (w870:T15)
        n301 = call <vilib>:"Add State(s) to Queue__JKI_lib_State_Machine.vi"("State(s) in (\"\")"=w876) -> ("States Out"=w875:string)  [unwired: 14 in]
      }
      frame "Data: Cleanup" {
        n302 = Unbundle By Name(w878) -> ("Core.Current VI Reference"=w881:refnum<vi>)
        n303 = Close Reference(reference=w881, error in (no error)=w880) -> (error out=w879:errorcluster)
        n304 = call <vilib>:"Add State(s) to Queue__JKI_lib_State_Machine.vi"("State(s) in (\"\")"=w883) -> ("States Out"=w882:string)  [unwired: 14 in]
      }
      frame "---------- UI ----------" {
        n305 = call <vilib>:"Add State(s) to Queue__JKI_lib_State_Machine.vi"("State(s) in (\"\")"=w888) -> ("States Out"=w887:string)  [unwired: 14 in]
      }
      frame "UI: Initialize" {
        n306 = Unbundle By Name(w891) -> ("Core.Current VI Reference"=w890:refnum<vi>)
        n307 = call <userlib>:"Fit VI window to Largest Dec__ogtk.vi"("error in (no error)"=w893, "VI Ref (calling VI)"=w890) -> ("error out"=w892:errorcluster, "dup VI Ref"=w889:refnum<vi>)  [unwired: 4 in]
        n308 = disable-structure shown="Disabled" {
          disable-tunnel: w889 -> [w898 _]
          frame Disabled {
            n309 = property class="VI"(reference=w898, "Front Panel.Title"="*VI Title*" ("Front Panel Window:Title")) -> ()  [unwired: 1 in, 2 out]
          }
          frame Enabled {
          }
        }
        n310 = call <vilib>:"Add State(s) to Queue__JKI_lib_State_Machine.vi"("State(s) in (\"\")"=w896) -> ("States Out"=w895:string)  [unwired: 14 in]
      }
      frame "UI: Cursor Set" {
        # "Argument"
        n311 = case shown="\"Idle\", Default" w900 {
          tunnel: w902 -> [w907 w909]
          tunnel: [w906 w908] -> w901
          frame "Idle", Default {
            n312 = call <vilib>:"Unset Busy.vi"("error in (no error)"=w907) -> ("error out"=w906:errorcluster)  [unwired: 10 in]
          }
          frame "Busy" {
            n313 = call <vilib>:"Set Busy.vi"("error in (no error)"=w909) -> ("error out"=w908:errorcluster)  [unwired: 9 in, 1 out]
          }
        }
        n314 = call <vilib>:"Add State(s) to Queue__JKI_lib_State_Machine.vi"("State(s) in (\"\")"=w905) -> ("States Out"=w904:string)  [unwired: 14 in]
      }
      frame "UI: Front Panel State" {
        # "Argument"
        n315 = Unbundle By Name(w913) -> ("Core.Current VI Reference"=w912:refnum<vi>)
        n316 = case shown="\"Close\"" w911 {
          tunnel: w915 -> [w921 w934]
          tunnel: [w923 w935] -> w914
          tunnel: w912 -> [w922 w932]
          frame "Open", Default {
            n317 = property class="VI"(reference=w922, error in=w921) -> (reference out=w919:refnum<vi>, error out=w920:errorcluster, "Front Panel.Open"=w918:bool)
            n318 = case shown="False" w918 {
              tunnel: [w926 w929] -> w923
              tunnel: w920 -> [w925 w929]
              tunnel: w919 -> [w924 _]
              frame False {
                n319 = invoke class="VI" method="FP.Open"(reference=w924, error in=w925, "Activate"=TRUE, "State"=T40."Standard") -> (error out=w926:errorcluster)  [unwired: 1 in, 4 out]
              }
              frame True {
              }
            }
          }
          frame "Close" {
            n320 = property class="VI"(reference=w932, error in=w934) -> (reference out=w931:refnum<vi>, error out=w933:errorcluster, "Front Panel.Open"=w930:bool)
            n321 = case shown="True" w930 {
              tunnel: [w936 w939] -> w935
              tunnel: w933 -> [w936 w938]
              tunnel: w931 -> [_ w937]
              frame False {
              }
              frame True {
                n322 = invoke class="VI" method="FP.Close"(reference=w937, error in=w938) -> (error out=w939:errorcluster)  [unwired: 1 in, 2 out]
              }
            }
          }
        }
        n323 = call <vilib>:"Add State(s) to Queue__JKI_lib_State_Machine.vi"("State(s) in (\"\")"=w917) -> ("States Out"=w916:string)  [unwired: 14 in]
      }
      frame "---------- Macro ----------" {
        n324 = call <vilib>:"Add State(s) to Queue__JKI_lib_State_Machine.vi"("State(s) in (\"\")"=w944) -> ("States Out"=w943:string)  [unwired: 14 in]
      }
      frame "Macro: Initialize" {
        n325 = call <vilib>:"Add State(s) to Queue__JKI_lib_State_Machine.vi"("State(s) in Front (\"\")"=w945, "State(s) in (\"\")"=w950) -> ("States Out"=w949:string)  [unwired: 13 in]
      }
      frame "Macro: Exit" {
        n326 = Unbundle By Name(w958) -> ("Core.Close Panel on Exit?"=w957:bool)
        n327 = Select(t="UI: Front Panel State >> Close", s=w957, f="") -> (s? t:f=w954:string)
        n328 = call <vilib>:"Add State(s) to Queue__JKI_lib_State_Machine.vi"("State(s) in (\"\")"=w954, "State(s) at Back (\"\")"=w951) -> ("States Out"=w953:string)  [unwired: 13 in]
        n329 = call <vilib>:"Add State(s) to Queue__JKI_lib_State_Machine.vi"("State(s) in Front (\"\")"=w953, "State(s) in (\"\")"=w961) -> ("States Out"=w960:string)  [unwired: 13 in]
      }
      frame "---------- Action ----------" {
        n330 = call <vilib>:"Add State(s) to Queue__JKI_lib_State_Machine.vi"("State(s) in (\"\")"=w966) -> ("States Out"=w965:string)  [unwired: 14 in]
      }
      frame "Action: StopProcessing" {
        n331 = Unbundle By Name(w973) -> ("Self Reference"=w969:refnum<class "Main.lvclass">, "ProcessingState"=w972:T14)  [unwired: 1 out]
        n332 = Bundle("ProcessingState"=w972, "Variant"=variant) -> (w974:T53)  [unwired: 1 in]
        n333 = call "Fire Private Event.vi"("error in (no error)"=w967, "vData"=w974, "PrivAsync"=PrivateAsynEv_Main--enum."PrivMain.UpdateProcessingState", "Main in"=w969) -> ("error out"=w968:errorcluster)  [unwired: 6 in, 1 out]
        n334 = call <vilib>:"Add State(s) to Queue__JKI_lib_State_Machine.vi"("State(s) in (\"\")"=w977) -> ("States Out"=w976:string)  [unwired: 14 in]
      }
      frame "Action: StartProcessing" {
        w978 = 4 ("dimension size")
        w1009 = T44 {"InverterInfo"={"Inverter ID"=""}, "ProcessInitParams"={"MinCurrThreshold"=1.5, "NumPF RdsToAvg"=10, "ESR alarm threshhold (%)"=200.0, "# readings to average"=40}}  # StartProcInitParams
        w1001 = T5 {"DUT ESR avg"=[], "DUT  PF avg"=[], "DUT  Power avg "=[], "DUT processed data"=[], "ESR alarm variables"=[], "Status data"=[], "CurrInverter"=[], "miscellaneous"=[], "DUT INVERTER data"=[]}  # Processing loop variables
        n335 = Unbundle By Name(w1011) -> ("ProcessingState"=w995:T14, "Self Reference"=w1007:refnum<class "Main.lvclass">, "vData"=w1010:variant)
        n336 = Variant To Data(error in=w996, type=w1009, Variant=w1010) -> (data=w1008:T44, error out=w1005:errorcluster)
        n337 = Unbundle By Name(w1008) -> ("InverterInfo"=w1002:T27, "InverterInfo.Inverter ID"=w990:string, "ProcessInitParams.MinCurrThreshold"=w984:dbl, "ProcessInitParams.NumPF RdsToAvg"=w999:i32, "ProcessInitParams.ESR alarm threshhold (%)"=w982:dbl, "ProcessInitParams.# readings to average"=w998:i32)
        n338 = Bundle By Name(cluster=T7 {"Inv 1 baseline ESR"=0.0, "Inv 1 over threshold?"=FALSE, "Alarm on?"=FALSE, "inv 1 esr chart range"=0.0, "inv 1 esr saved baseline"=0.0, "ESR alarm threshhold"=0.0} ("ESR alarm variables"), "ESR alarm threshhold"=w982) -> (w981:T7)
        n339 = Bundle By Name(cluster=T41 {"Inv. 1 on?"=FALSE, "Inv. 1 ESR over threshhold?"=FALSE, "Minimum current"=0.0} ("Status data"), "Minimum current"=w984) -> (w986:T41)
        n340 = Bundle By Name(cluster=T42 {"Inverter 1 ID"="", "Inverter 2 ID"="", "Packet count"=0, "Calibration"=0.0, "Calibration Gain"=0.0, "Calibration Offset"=0.0, "Calculated Total Power"=0.0, "Seconds"=0.0, "Last Tag Event"=0.0, "Tag Event Time"=0.0} ("miscellaneous"), "Inverter 1 ID"=w990) -> (w989:T42)
        n341 = property class="Main.lvclass"(reference=w1007, error in=w1005, "Accessors:InverterInfo*"=w1002) -> (reference out=w1006:refnum<class "Main.lvclass">, error out=w1004:errorcluster, "Accessors:CurrInverter*"=w979:T8[])
        n342 = Initialize Array(w986, w978) -> (w985:T54)
        n343 = Initialize Array(w989, w978) -> (w988:T55)
        n344 = Initialize Array(w981, w978) -> (w980:T7[])
        n345 = Bundle By Name(cluster=w1001, "CurrInverter"=w979, "miscellaneous"=w988, "Status data"=w985, "ESR alarm variables"=w980) -> (w1000:T5)
        n346 = call "initialize averaging variables.vi"("# of  power factor reads to avg"=w998, "error in (no error)"=w1004, "# of ESR reads to  average"=w999, "Processing loop variables"=w1000) -> ("error out"=w1003:errorcluster, "Processing loop variables out"=w993:T5)  [unwired: 6 in]
        n347 = To Variant(anything=w993) -> (Variant=w992:variant)
        n348 = Bundle("ProcessingState"=w995, "Variant"=w992) -> (w994:T53)  [unwired: 1 in]
        n349 = call "Fire Private Event.vi"("error in (no error)"=w1003, "vData"=w994, "PrivAsync"=PrivateAsynEv_Main--enum."PrivMain.UpdateProcessingState", "Main in"=w1006) -> ("error out"=w997:errorcluster)  [unwired: 6 in, 1 out]
        n350 = call <vilib>:"Add State(s) to Queue__JKI_lib_State_Machine.vi"("State(s) in (\"\")"=w1015) -> ("States Out"=w1014:string)  [unwired: 14 in]
      }
      frame "Action: Wait" {
        n351 = Scan From String(format string="%d", input string=w1016, error in=w1018, default 1=u32 0) -> (error out=w1022:errorcluster, output 1=w1021:u32)  [unwired: 1 in, 2 out]
        n352 = call <userlib>:"Wait (ms)__ogtk.vi"("error in (no error)"=w1022, "milliseconds to wait"=w1021) -> ("error out"=w1017:errorcluster)  [unwired: 8 in, 1 out]
        n353 = call <vilib>:"Add State(s) to Queue__JKI_lib_State_Machine.vi"("State(s) in (\"\")"=w1026) -> ("States Out"=w1025:string)  [unwired: 14 in]
      }
      frame "Action: Terminate AsyncLoop" {
        n354 = Unbundle By Name(w1033) -> ("SMQ"=w1037:refnum<queue>)
        n355 = Unbundle By Name(w1033) -> ("Self Reference"=w1032:refnum<class "Main.lvclass">)
        n356 = Flush Queue(queue=w1037) -> (queue out=w1036:refnum<queue>)  [unwired: 1 in, 2 out]
        n357 = call <vilib>:"Add State to Queue with vData.vi"("queue in"=w1036, "state in"="Macro: Exit", "error in"=w1034) -> ("error out"=w1031:errorcluster)  [unwired: 9 in, 3 out]
        n358 = call "Fire Private Event.vi"("error in (no error)"=w1031, "PrivAsync"=PrivateAsynEv_Main--enum."PrivMain.Stop&Terminate", "Main in"=w1032) -> ("error out"=w1030:errorcluster)  [unwired: 7 in, 1 out]
        n359 = call <userlib>:"Wait (ms)__ogtk.vi"("error in (no error)"=w1030, "milliseconds to wait"=u32 1000) -> ("error out"=w1028:errorcluster)  [unwired: 8 in, 1 out]
        n360 = call <vilib>:"Add State(s) to Queue__JKI_lib_State_Machine.vi"("State(s) in (\"\")"=w1040) -> ("States Out"=w1039:string)  [unwired: 14 in]
      }
    }
  }
  n361 = Merge Errors(w6, w5) -> ()  [unwired: 1 out]
